vi "MU Library Demo.vi"() -> ()   [LabVIEW 2017]
uses:
  enums/MU_Interface.ctl
  enums/MU_ConfigData.ctl
  enums/MU_Param.ctl
  enums/MU_WriteVerify.ctl
  enums/MU_E2PArea.ctl
  enums/MU_Command.ctl
  enums/MU_ErrorType.ctl
  enums/MU_InterfaceInfo.ctl
  enums/MU_Error.ctl
  enums/MU_Unit.ctl
  enums/MU_AdjustmentMessage.ctl
  enums/MU_BissProfile.ctl
  Controls/MU_Functions.ctl
  handles/CalibrationHandle.ctl
  handles/CalibrationAnalyzeResultHandle.ctl
  handles/mtSyncHandle.ctl
  handles/mtSyncAnalyzeResultHandle.ctl
  MU_3SL_interface.lvlib
panel:
  in  "Stop Button":bool
  in  "TabControl":T1(tab)
  in  "MU_InterfaceInfo":T2
  in  "MU_Interface":T3
  in  "MU_Close":bool
  in  "MU_GetInterface":bool
  in  "MU_SetInterface":bool
  in  "MU_Open":bool
  out "MU_Interface":T3
  in  "MU_GetInterfaceInfo":bool caption="MU_GetInterface"
  out "information":string
  in  "interfaceOption":string
  in  "MU_ConfigData":T4
  in  "MU_ConfigData":T4
  in  "MU_GetConfig":bool
  in  "MU_SetConfig":bool
  in  "value":u32 format="0x%02x"
  out "value":u32 format="0x%02x"
  in  "MU_Initialize":bool caption="MU_GetConfig"
  in  "MU_SwitchToBiSS":bool caption="MU_GetConfig"
  out "modea":u32 format="0x%02x"
  out "modeb":u32 format="0x%02x"
  in  "MU_SwitchToBiSS_Ex":bool caption="MU_GetConfig"
  out "modea":u32 format="0x%02x"
  in  "MU_UseRevision":bool caption="MU_GetConfig"
  in  "revisionId":u32 format="0x%02x"
  in  "MU_ReadChipRevision":bool caption="MU_GetConfig"
  out "revisionId":u32 format="0x%02x"
  in  "MU_ValueOfUsedRevision":bool caption="MU_GetConfig"
  out "revisionId":u32 format="0x%02x"
  out "switched":bool
  out "isInRevision":bool
  in  "MU_Command":T5
  in  "MU_E2PArea":T6
  in  "MU_WriteVerifyEnum 2":T7 caption="MU_WriteVerify"
  in  "MU_WriteParams":bool
  in  "MU_SetParam":bool
  in  "MU_GetParam":bool
  in  "MU_ReadParams":bool
  in  "MU_ParamEnum 3":T8 caption="MU_Param"
  in  "ulValue":u64 caption="value" format="0x%08x"
  in  "MU_ParamEnum 3":T8 caption="MU_Param"
  out "pulValue":u64 caption="value" format="0x%08x"
  in  "MU_ReadStatus":bool caption="MU_GetDLLVersion"
  in  "MU_WriteEeprom":bool caption="MU_WriteParams"
  in  "MU_WriteCmdRegister":bool caption="MU_WriteParams"
  in  "MU_WriteSwitchCommand":bool caption="MU_WriteParams"
  in  "modeaNew":u32 format="0x%02x"
  in  "rplNew":u32 format="0x%02x"
  in  "MU_ReadGain":bool caption="MU_GetDLLVersion"
  in  "verify":bool
  out "valid":bool[](array[boolean])
  in  "MU_IsParameterAvailableInUsedRevision":bool caption="MU_GetParam"
  in  "MU_ParamEnum 4":T8 caption="MU_Param"
  in  "MU_ReadSens":bool caption="MU_WriteParams"
  out "data":T9 {"mt" format="0x%02x"; "st" format="0x%02x"; "err" format="0x%02x"; "warn" format="0x%02x"; "rawMaster" format="0x%02x"; "rawNonius" format="0x%02x"}
  out "noniusRawData":u16[](array[numeric])
  out "masterRawData":u16[](array[numeric])
  in  "clockFrequency":dbl
  in  "frameCycleTime":dbl
  in  "SlaveID":u32
  in  "numberOfSamples":u64
  in  "MU_acquireRawData":bool caption="MU_WriteParams"
  in  "MU_activateCalibrationConfig":bool caption="MU_WriteParams"
  in  "MU_deactivateCalibrationConfig":bool caption="MU_WriteParams"
  in  "MU_Get Calibration":bool caption="MU_WriteParams"
  in  "MU_Set Calibration":bool caption="MU_WriteParams"
  in  "MU_CreateCalibration":bool caption="MU_WriteParams"
  in  "revisionCode":u8 format="%.0x"
  in  "MU_Calibration_delete":bool caption="MU_WriteParams"
  in  "NumberOfMasterPeriods (0=autodetect)":u32
  in  "MU_Calibration_preconfigureNumberOfMasterPeriods":bool caption="MU_WriteParams"
  out "Return value":bool
  in  "noniusTrackRawData":u16[](array[numeric])
  in  "masterTrackRawData":u16[](array[numeric])
  in  "numberOfRawDataSamples":u64
  in  "MU_Calibration_analyzeRawData":bool caption="MU_WriteParams"
  in  "MU_CalibrationAnalyzeResult_delete":bool caption="MU_WriteParams"
  out "size":u64
  in  "MU_Calibration_getAnalyzeResultLog":bool caption="MU_WriteParams"
  in  "logDestSize":u64=1024
  out "logDest":string
  in  "MU_AdjustmentLogLevel":T10 format="0x%02x"
  in  "MU_Calibration_getOptimizedNoniusTrackOffsetTableBaseOnly":bool caption="MU_WriteParams"
  out "optimizedNoniusTrackOffsetTableBaseOnly":cluster{"spoBase":i8, "spoN":i8[]}
  in  "MU_Calibration_numberOfAcquiredNoniusPeriods":bool caption="MU_WriteParams"
  out "acquiredNoniusPeriods":dbl
  in  "MU_Calibration_getRelativeMasterTrackAdjustments":bool caption="MU_WriteParams"
  out "MU_Calibration_RelativeAnalogTrackAdjustments_Master":T11
  in  "MU_Calibration_getRelativeNoniusTrackAdjustments":bool caption="MU_WriteParams"
  out "MU_Calibration_RelativeAnalogTrackAdjustments_Nonius":T11
  in  "MU_Calibration_numberOfCalculatedMasterPeriods":bool caption="MU_WriteParams"
  out "CalculatedMasterPeriods":i32
  in  "MU_Calibration_isAnalogAnalysesValid":bool caption="MU_WriteParams"
  out "isAnalogAnalysesValid":bool
  in  "MU_Calibration_isNoniusAnalysesValid":bool caption="MU_WriteParams"
  out "isNoniusAnalysesValid":bool
  out "NumberOfRevolutions":dbl
  in  "MU_Calibration_numberOfRevolutions":bool caption="MU_WriteParams"
  in  "MU_Calibration_numberOfAcquiredMasterPeriods":bool caption="MU_WriteParams"
  out "acquiredMasterPeriods":dbl
  in  "MU_Calibration_minimalNumberOfSamplesPerMasterPeriod":bool caption="MU_WriteParams"
  out "minimalNumberOfSamplesPerMasterPeriod":dbl
  in  "MU_Calibration_getOptimizedNoniusTrackOffsetTable":bool caption="MU_WriteParams"
  out "optimizedNoniusTrackOffsetTable":cluster{"spoBase":i8, "spoN":i8[]}
  in  "MU_Calibration_noniusTrackOffsetCurve":bool caption="MU_WriteParams"
  out "TrackOffset":i32[](array[numeric])
  in  "MU_Calibration_noniusPhaseMargin":bool caption="MU_WriteParams"
  out "PhaseMargin":i32[](array[numeric])
  out "PhaseError":i32[](array[numeric])
  in  "MU_Calibration_noniusPhaseError":bool caption="MU_WriteParams"
  out "Return Value":u64
  out "SingleturnPosition":dbl[](array[numeric])
  in  "Continuous":bool
  in  "MU_Calibration_calculateNoniusPosition":bool caption="MU_WriteParams"
  in  "MU_Unit":T12 format="0x%02x"
  out "NoniusPhaseMarginMin":i32
  in  "MU_Calibration_noniusPhaseMarginMin":bool caption="MU_WriteParams"
  in  "MU_Calibration_noniusPhaseMarginMax":bool caption="MU_WriteParams"
  out "NoniusPhaseMarginMax":i32
  in  "MU_Calibration_noniusPhaseRangeLimit":bool caption="MU_WriteParams"
  in  "MU_Calibration_noniusUpperPhaseMargin":bool caption="MU_WriteParams"
  in  "MU_Calibration_NoniusLowerPhaseMargin":bool caption="MU_WriteParams"
  out "noniusLowerPhaseMargin":dbl
  out "noniusUpperPhaseMargin":dbl
  out "noniusPhaseRangeLimit":i32
  out "NumberOfNoniusCurveSamples":u64
  in  "MU_Calibration_numberOfNoniusCurveSamples":bool caption="MU_WriteParams"
  in  "optimizedNoniusTrackOffsetTable":cluster{"spoBase":i8, "spoN":i8[]}={"spoBase"=0, "spoN"=[0, 0, 0, 0, 0, 0, 0, 0, 0, 0, 0, 0, 0, 0, 0, 0]}
  in  "MU_Calibration_setCurrentNoniusTrackOffsetTable":bool caption="MU_WriteParams"
  in  "noniusAdjustments":T13 {"phaseRange" format="%.0x"; "phase" format="%.0x"; "cosineOffset" format="%.0x"; "sineOffset" format="%.0x"; "cosineGain" format="%.0x"}
  in  "masterAdjustments":T13 {"phaseRange" format="%.0x"; "phase" format="%.0x"; "cosineOffset" format="%.0x"; "sineOffset" format="%.0x"; "cosineGain" format="%.0x"}
  in  "MU_Calibration_setCurrentAnalogTrackAdjustments":bool caption="MU_WriteParams"
  out "function return":bool
  in  "MU_Calibration_adjustAnalogByAnalyzeResult":bool caption="MU_WriteParams"
  in  "MU_AdjustmentLogLevel":T10 format="0x%02x"
  out "Result":bool
  out "adjustMessage":string
  in  "adjustmentMessageBufferSize":u64=1024
  in  "MU_Calibration_isAnalogAnalyzeResultAdjustable":bool caption="MU_WriteParams"
  in  "MU_Calibration_getAnalogMasterTrackAdjustments":bool caption="MU_WriteParams"
  out "masterAdjustments":T13 {"phaseRange" format="%.0x"; "phase" format="%.0x"; "cosineOffset" format="%.0x"; "sineOffset" format="%.0x"; "cosineGain" format="%.0x"}
  in  "MU_Calibration_getAnalogNoniusTrackAdjustments":bool caption="MU_WriteParams"
  out "noniusAdjustments":T13 {"phaseRange" format="%.0x"; "phase" format="%.0x"; "cosineOffset" format="%.0x"; "sineOffset" format="%.0x"; "cosineGain" format="%.0x"}
  in  "MU_Calibration_getNoniusTrackOffsetTable":bool caption="MU_WriteParams"
  out "NoniusTrackOffsetTable":cluster{"spoBase":i8, "spoN":i8[]}
  out "noniusTrackOffsetTable":cluster{"spoBase":i8, "spoN":i8[]}
  in  "noniusTrackOffsetTableParameters":cluster{"spoBase":u8, "spoN":u8[]}={"spoBase"=0, "spoN"=[0, 0, 0, 0, 0, 0, 0, 0, 0, 0, 0, 0, 0, 0, 0, 0]}
  out "noniusTrackOffsetTableParameters":cluster{"spoBase":u8, "spoN":u8[]}
  in  "noniusTrackOffsetTable":cluster{"spoBase":i8, "spoN":i8[]}={"spoBase"=0, "spoN"=[0, 0, 0, 0, 0, 0, 0, 0, 0, 0, 0, 0, 0, 0, 0, 0]}
  in  "MU_getNoniusTrackOffsetTableParameters":bool caption="MU_WriteParams"
  in  "MU_getNoniusTrackOffsetTableByParameters":bool caption="MU_WriteParams"
  out "nextClockFrequency":dbl format="%#_6f"
  in  "clockFrequency_hz":dbl format="%#_6f"
  in  "MU_Interface_nextPossibleClockFreq":bool caption="MU_WriteParams"
  in  "frameCycleTime_s":dbl format="%#_6f"
  in  "MU_Interface_nextPossibleFrameCycleTime":bool caption="MU_WriteParams"
  out "nextFrameCycleTime":dbl format="%#_6f"
  out "nearestFrameCycleTime":dbl format="%#_6f"
  in  "frameCycleTime_s":dbl format="%#_6f"
  in  "MU_Interface_nearestPossibleFrameCycleTime":bool caption="MU_WriteParams"
  out "nearestClockFrequency":dbl format="%#_6f"
  in  "clockFrequency_hz":dbl format="%#_6f"
  in  "MU_Interface_nearestPossibleClockFreq":bool caption="MU_WriteParams"
  in  "MU_Interface":T3 format="0x%02x"
  in  "MU_Interface":T3 format="0x%02x"
  in  "MU_Interface":T3 format="0x%02x"
  in  "MU_Interface":T3 format="0x%02x"
  in  "MU_acquire3TrackMtSyncData":bool caption="MU_WriteParams"
  in  "Samples":u64
  out "SyncData":T14(array[cluster])
  in  "MU_acquireMtSyncData":bool caption="MU_WriteParams"
  in  "Samples":u64
  out "data":T15(array[cluster])
  in  "MU_activateMtSyncConfig":bool caption="MU_WriteParams"
  in  "MU_deactivateMtSyncConfig":bool caption="MU_WriteParams"
  in  "MU_activate3TrackMtSyncConfig":bool caption="MU_WriteParams"
  in  "MU_deactivate3TrackMtSyncConfig":bool caption="MU_WriteParams"
  in  "MU_MtSync_calculatePosition":bool caption="MU_WriteParams"
  in  "SyncData":T15(array[cluster])
  out "MT_Position":dbl[](array[numeric])
  in  "Samples":u64
  in  "MtTrackOffset":u8
  in  "Calibration Unit":u32
  in  "resolution":u64
  in  "Continuous (F)":bool
  in  "MU_getMtSync":bool caption="MU_WriteParams"
  in  "MU_updateMtSync":bool caption="MU_WriteParams"
  in  "mtMovementIsReverse":bool
  in  "nMtSyncBits":u64
  in  "MU_createMtSync":bool caption="MU_WriteParams"
  in  "MU_MtSync_delete":bool caption="MU_WriteParams"
  in  "numberOfSamples":u64
  in  "data":T15(array[cluster])
  in  "MU_MtSync_analyzeData":bool caption="MU_WriteParams"
  in  "MU_MtAnalyzeResult_delete":bool caption="MU_WriteParams"
  out "optimalSpoMt":u8
  in  "MU_MtAnalyzeResult_optimalSpoMt":bool caption="MU_WriteParams"
  in  "MtTrackOffset":u8
  out "MT_OffsetError":dbl[](array[numeric])
  in  "MU_MtAnalyzeResult_calculateOffsetError":bool caption="MU_WriteParams"
  in  "Samples":u64
  out "Return Value":u64
  out "UpperOffsetErrorMargin":dbl
  in  "MtTrackOffset":u8
  in  "MU_MtAnalyzeResult_upperOffsetErrorMargin":bool caption="MU_WriteParams"
  in  "MtTrackOffset":u8
  out "LowerOffsetErrorMargin":dbl
  in  "MU_MtAnalyzeResult_lowerOffsetErrorMargin":bool caption="MU_WriteParams"
  out "OffsetErrorRangeLimit":dbl
  in  "MU_MtAnalyzeResult_offsetErrorRangeLimit":bool caption="MU_WriteParams"
  out "MinOffsetError":dbl
  in  "MtTrackOffset":u8
  in  "MU_MtAnalyzeResult_minOffsetError":bool caption="MU_WriteParams"
  in  "MtTrackOffset":u8
  out "MaxOffsetError":dbl
  in  "MU_MtAnalyzeResult_maxOffsetError":bool caption="MU_WriteParams"
  in  "MU_BissProfile":T16 format="0x%02x"
  in  "MU_generateBissProfileId":bool caption="MU_GetDLLVersion"
  in  "MU_generateBissIdentifier":bool caption="MU_GetDLLVersion"
  out "MU_Error":T17
  in  "MU_SaveParams":bool
  in  "MU_LoadParams":bool
  in  "data":u32 format="0x%02x"
  in  "MU_SPIActivate":bool caption="MU_GetDLLVersion"
  in  "MU_GetLastError":bool caption="MU_GetDLLVersion"
  out "lastErrorText":string
  out "MU_ErrorType":T18
  in  "MU_CalcPres_POS":bool caption="MU_GetDLLVersion"
  in  "value":u64 format="0x%08x"
  in  "MU_GetPres_POS":bool caption="MU_GetDLLVersion"
  out "value":u64 format="0x%08x"
  in  "MU_WriteVerifyEnum":T7 caption="MU_WriteVerify"
  out "modea":u32 format="0x%02x"
  in  "MU_EnableGetMT":bool caption="MU_GetDLLVersion"
  in  "MU_DisableGetMT":bool caption="MU_GetDLLVersion"
  in  "pcCfgFilename":path caption="filepath"
  in  "pcCfgFilename 2":path caption="filepath"
  out "switched":bool
  in  "MU_ReadChipRevisionOfParameterFile":bool caption="MU_SaveParams"
  in  "pcCfgFilename 5":path caption="filepath"
  out "revisionCode":u32 format="0x%02x"
  out "bissProfileId":u16 format="%.0x"
  out "deviceID":u64 format="%.0x"
  out "mfgID":u16 format="%.0x"
  out "versionBuild":u16 format="%.0x"
  out "versionPatch":u16 format="%.0x"
  out "versionMinor":u16 format="%.0x"
  out "versionMajor":u16 format="%.0x"
  out "versionSuffixString":string
  in  "MU_GetVersionSuffixString":bool caption="MU_WriteParams"
  in  "MU_GetVersionBuild":bool caption="MU_WriteParams"
  in  "MU_GetVersionPatch":bool caption="MU_WriteParams"
  in  "MU_GetVersionMinor":bool caption="MU_WriteParams"
  in  "MU_GetVersionMajor":bool caption="MU_WriteParams"
  out "versionString":string
  in  "MU_GetVersionString":bool caption="MU_WriteParams"
  out "version":u32[](array[numeric]) format="0x%02x"
  in  "MU_GetDLLVersion":bool
  in  "MU_GetRegister":bool
  in  "MU_SetRegister":bool
  in  "address":u32 format="0x%02x"
  in  "ulValue":u32 caption="value" format="0x%02x"
  in  "MU_WriteVerifyEnum 2":T7 caption="MU_WriteVerify"
  in  "ulAdr":u32 caption="address" format="0x%02x"
  out "pulValue":u32 caption="value" format="0x%02x"
  in  "MU_WriteRegister":bool caption="MU_GetRegister"
  in  "address":u32 format="0x%02x"
  in  "count":u32 format="0x%02x"
  in  "values":u32[](array[numeric]) format="0x%02x"
  in  "MU_ReadRegister":bool caption="MU_GetRegister"
  in  "address":u32 format="0x%02x"
  in  "count":u32 format="0x%02x"
  out "values":u32[](array[numeric]) format="0x%02x"
  in  "MU_SaveRegister":bool caption="MU_SaveParams"
  in  "address":u32 format="0x%02x"
  in  "count":u32 format="0x%02x"
  in  "values":u32[](array[numeric]) format="0x%02x"
  in  "MU_LoadRegister":bool caption="MU_LoadParams"
  in  "count":u32 format="0x%02x"
  in  "address":u32 format="0x%02x"
  out "values":u32[](array[numeric]) format="0x%02x"
  in  "values":u32[](array[numeric]) format="0x%02x"
  in  "count":u32 format="0x%02x"
  in  "address":u32 format="0x%02x"
  in  "MU_WriteRegisterSSI":bool caption="MU_GetRegister"
  in  "pcFilename":path caption="filepath"
  in  "pcCfgFilename 3":path caption="filepath"
  in  "MU_WriteRegister_I2C":bool caption="MU_GetDLLVersion"
  in  "values":u32[](array[numeric]) format="0x%02x"
  in  "MU_WriteRegister_I2C_Ex":bool caption="MU_GetDLLVersion"
  in  "values":u32[](array[numeric]) format="0x%02x"
  in  "i2cSlaveAddress":u32 format="0x%02x"
  in  "registerCount":u32 format="0x%02x"
  in  "registerCount":u32 format="0x%02x"
  in  "registerAddress":u32 format="0x%02x"
  in  "i2cSlaveAddress":u32 format="0x%02x"
  in  "MU_ReadRegister_I2C":bool caption="MU_GetDLLVersion"
  out "values":u32[](array[numeric]) format="0x%02x"
  in  "i2cSlaveAddress":u32 format="0x%02x"
  in  "registerCount":u32 format="0x%02x"
  in  "registerAddress":u32 format="0x%02x"
  in  "MU_LoadRegisterEx":bool caption="MU_GetDLLVersion"
  out "values":u32[](array[numeric]) format="0x%02x"
  in  "registerCount":u32 format="0x%02x"
  in  "MU_SaveRegisterEx":bool caption="MU_GetDLLVersion"
  in  "values":u32[](array[numeric]) format="0x%02x"
  in  "registerCount":u32 format="0x%02x"
  in  "registerAddress":u32 format="0x%02x"
  in  "pcCfgFilename 4":path caption="filepath"
  in  "pcFilename 2":path caption="filepath"
  in  "valid":bool[](array[boolean])
  out "valid":bool[](array[boolean])
  # "iC-MU Series Library Demo"
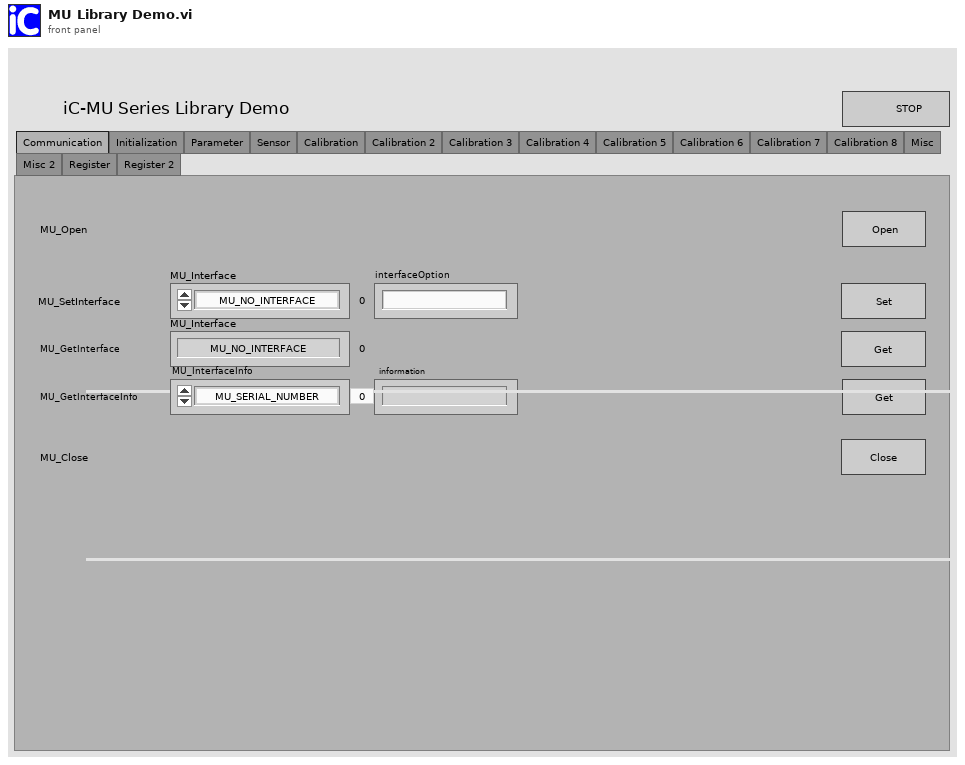
[diagram p1: front panel]
types:
  T1 = enum32{"Communication", "Initialization", "Parameter", "Sensor", "Calibration", "Calibration 2", "Calibration 3", "Calibration 4", "Calibration 5", "Calibration 6", "Calibration 7", "Calibration 8", "Misc", "Misc 2", "Register", "Register 2"}
  T2 = typedef "MU_3SL_interface.lvlib/MU_InterfaceInfo.ctl" = enum32{"MU_SERIAL_NUMBER", "MU_DRIVER_VERSION"}
  T3 = typedef "MU_3SL_interface.lvlib/MU_Interface.ctl" = enum32{"MU_NO_INTERFACE", "MU_MB3U_SPI", "MU_MB3U_BISS", "MU_MB4U", "MU_MB5U"}
  T4 = typedef "MU_3SL_interface.lvlib/MU_ConfigData.ctl" = enum32{"MU_RESERVED0", "MU_FREQ_SPI", "MU_MASTERVER", "MU_MASTERREV", "MU_SLAVE_ID", "MU_FREQ_SCD", "MU_CLKENI", "MU_FREQ_AGS", "MU_SLAVE_COUNT", "MU_START_CONTROL_FRAME", "MU_REG_END", "MU_FREQ_SSI", "MU_READ_STATUS_ENABLE", "MU_USB_PERFORMANCE", "MU_READ_GAIN_ENABLE", "MU_BP", "MU_UPDATE_BISSID_ENABLE", "MU_ENABLE_TTL"}
  T5 = typedef "MU_3SL_interface.lvlib/MU_Command.ctl" = enum32{"MU_CMD_NO_FUNCTION", "MU_CMD_WRITE_ALL", "MU_CMD_WRITE_OFF", "MU_CMD_ABS_RESET", "MU_CMD_NON_VER", "MU_CMD_MT_RESET", "MU_CMD_MT_VER", "MU_CMD_SOFT_RESET", "MU_CMD_SOFT_PRES", "MU_CMD_SOFT_E2P_PRES", "MU_CMD_I2C_COM", "MU_CMD_EVENT_COUNT", "MU_CMD_SWITCH", "MU_CMD_CRC_VER", "MU_CMD_CRC_CALC", "MU_CMD_SET_MTC", "MU_CMD_RES_MTC", "MU_CMD_RESERVED0", "MU_CMD_MODEA_SPI", "MU_CMD_ROT_POS", "MU_CMD_ROT_POS_E2P"}
  T6 = typedef "MU_3SL_interface.lvlib/MU_E2PArea.ctl" = enum32{"MU_E2P_CFG"}
  T7 = typedef "MU_3SL_interface.lvlib/MU_WriteVerify.ctl" = enum32{"MU_SETONLY", "MU_WRITE", "MU_VERIFY"}
  T8 = typedef "MU_3SL_interface.lvlib/MU_Param.ctl" = enum32{"MU_GF_M", "MU_GC_M", "MU_GX_M", "MU_VOSS_M", "MU_VOSC_M", "MU_PH_M", "MU_PHR_M", "MU_CIBM", "MU_ENAC", "MU_GF_N", "MU_GC_N", "MU_GX_N", "MU_VOSS_N", "MU_VOSC_N", "MU_PH_N", "MU_PHR_N", "MU_MODEA", "MU_NTOA", "MU_MODEB", "MU_CFGEW", "MU_EMTD", "MU_ACRM_RES", "MU_NCHK_NON", "MU_NCHK_CRC", "MU_ACC_STAT", "MU_FILT", "MU_LIN", "MU_ESSI_MT", "MU_ROT_MT", "MU_MPC", "MU_SPO_MT", "MU_MODE_MT", "MU_SBL_MT", "MU_CHK_MT", "MU_GET_MT", "MU_OUT_MSB", "MU_OUT_ZERO", "MU_OUT_LSB", "MU_MODE_ST", "MU_RSSI", "MU_GSSI", "MU_RESABZ", "MU_FRQAB", "MU_ENIF_AUTO", "MU_SS_AB", "MU_ROT_ALL", "MU_INV_Z", "MU_INV_B", "MU_INV_A", "MU_PP60UVW", "MU_CHYS_AB", "MU_LENZ", "MU_PPUVW", "MU_RPL", "MU_TEST", "MU_ROT_POS", "MU_OFF_ABZ", "MU_OFF_POS", "MU_OFF_COM", "MU_PA0_CONF", "MU_AFGAIN_M", "MU_ACGAIN_M", "MU_AFGAIN_N", "MU_ACGAIN_N", "MU_EDSBANK", "MU_PROFILE_ID", "MU_SERIAL", "MU_OFF_UVW", "MU_PRES_POS", "MU_SPO_BASE", "MU_SPO_0", "MU_SPO_1", "MU_SPO_2", "MU_SPO_3", "MU_SPO_4", "MU_SPO_5", "MU_SPO_6", "MU_SPO_7", "MU_SPO_8", "MU_SPO_9", "MU_SPO_10", "MU_SPO_11", "MU_SPO_12", "MU_SPO_13", "MU_SPO_14", "MU_SPO_15", "MU_RPL_RESET", "MU_I2C_DEV_START", "MU_I2C_RAM_START", "MU_I2C_RAM_END", "MU_I2C_DEVID", "MU_I2C_RETRY", "MU_HARD_REV", "MU_DEV_ID0", "MU_DEV_ID1", "MU_DEV_ID2", "MU_DEV_ID3", "MU_DEV_ID4", "MU_DEV_ID5", "MU_MFG_ID0", "MU_MFG_ID1", "MU_CRC16", "MU_CRC8", "MU_AM_MIN", "MU_AM_MAX", "MU_AN_MIN", "MU_AN_MAX", "MU_STUP", "MU_CMD_EXE", "MU_FRQ_CNV", "MU_FRQ_ABZ", "MU_NON_CTR", "MU_MT_CTR", "MU_MT_ERR", "MU_EPR_ERR", "MU_CRC_ERR"}
  T9 = cluster{"mt":u32, "st":u32, "err":u32, "warn":u32, "rawMaster":u32, "rawNonius":u32}
  T10 = typedef "MU_3SL_interface.lvlib/MU_AdjustmentMessage.ctl" = enum32{"MU_LOG_NONE", "MU_LOG_ERRORS", "MU_LOG_WARNINGS", "MU_LOG_ERRORS_WARNINGS", "MU_LOG_NOTE", "MU_LOG_ERRORS_NOTE", "MU_LOG_WARNINGS_NOTE", "MU_LOG_ALL"}
  T11 = cluster{"cosineGain_lsb":dbl, "sineOffset_lsb":dbl, "cosineOffset_lsb":dbl, "phase_lsb":dbl}
  T12 = typedef "MU_3SL_interface.lvlib/MU_Unit.ctl" = enum32{"MU_RESOLUTION", "MU_TURN", "MU_DEGREE", "MU_RAD"}
  T13 = cluster{"cosineGain":u8, "sineOffset":u8, "cosineOffset":u8, "phase":u8, "phaseRange":u8}
  T14 = cluster{"SingleTurnPosition":u32, "InternalSingleTurnPosition":u32, "NormalizedExternalMultiTurnSyncBits":u32, "NormalizedInternalMultiTurnSyncBits":u32, "externalMultiTurnPosition":u32, "multiTurnPosition":u32, "scdDataH":u64}[]
  T15 = cluster{"SingleTurnPosition":u32, "InternalSingleTurnPosition":u32, "NormalizedExternalMultiTurnSyncBits":u32, "NormalizedInternalMultiTurnSyncBits":u32, "externalMultiTurnPosition":u32, "multiTurnPosition":u32, "scdData":u64}[]
  T16 = typedef "MU_3SL_interface.lvlib/MU_BissProfile.ctl" = enum32{"MU_BISS_PROFILE_BP1", "MU_BISS_PROFILE_BP3"}
  T17 = typedef "MU_3SL_interface.lvlib/MU_Error.ctl" = enum32{"MU_OK", "MU_INVALID_HANDLE", "MU_INTERFACEDRIVER_NOT_FOUND", "MU_INTERFACE_NOT_FOUND", "MU_INVALID_INTERFACE", "MU_NO_INTERFACE_SELECTED", "MU_INVALID_PARAMETER", "MU_INVALID_ADDRESS", "MU_INVALID_VALUE", "MU_USB_ERROR", "MU_FILE_NOT_FOUND", "MU_INVALID_FILE", "MU_SPI_ERROR", "MU_SPI_DISMISS", "MU_SPI_FAIL", "MU_SPI_BUSY_TIMEOUT", "MU_VERIFY_FAILED", "MU_MASTERCOMM_FAILED", "MU_BISSCOMM_FAILED", "MU_INVALID_BISSMASTER", "MU_USB_HIGHSPEED_WARNING", "MU_FAST_ROTATION", "MU_SLOW_ROTATION", "MU_FILE_ACCESS_DENIED", "MU_READPARAM_SSI", "MU_SSIRING_ERROR", "MU_SEMI_ROTATION", "MU_BISS_REGERROR", "MU_INTERNAL_CALIB_ERROR", "MU_INVALID_CONFIGURATION", "MU_CALIBRATION_FAILED", "MU_ACQUISITION_FAILED", "MU_GAIN_LIMIT", "MU_OFFSET_LIMIT", "MU_PHASE_LIMIT", "MU_BAD_CAL_DATA", "MU_I2C_COMM_FAILED", "MU_USB_DATA_LOSS", "MU_MT_SYNC_FAILED", "MU_UNKNOWN_ERROR", "MU_UNKNOWN_REVISION", "MU_UNSUPPORTED_REVISION", "MU_UNKNOWN_PARAMETER", "MU_PARAMETER_NOT_IN_REVISION", "MU_REVISION_NOT_SET", "MU_UNSUPPORTED_CHIP", "MU_CONTRADICTORY_REVISIONS", "MU_FRAME_RATE_NOT_SUPPORTED", "MU_CLOCK_FREQUENCY_NOT_SUPPORTED", "MU_FRAME_CYCLE_TIME_TO_SHORT", "MU_NO_BISS_PROFILE_ID"}
  T18 = typedef "MU_3SL_interface.lvlib/MU_ErrorType.ctl" = enum32{"MU_NONE", "MU_HINT", "MU_WARNING", "MU_PROGRAMMING_ERROR", "MU_OPERATING_ERROR", "MU_COMMUNICATION_ERROR"}
  T19 = typedef "MU_3SL_interface.lvlib/mtSyncAnalyzeResultHandle.ctl" = u64
  T20 = typedef "MU_3SL_interface.lvlib/mtSyncHandle.ctl" = u64
  T21 = typedef "MU_3SL_interface.lvlib/CalibrationAnalyzeResultHandle.ctl" = u64
  T22 = typedef "MU_3SL_interface.lvlib/CalibrationHandle.ctl" = u64
  T23 = typedef "MU_Functions.ctl" = enum16{"Start Demo", "Open", "Close", "Set Interface", "Get Interface", "Set Config", "Get Config", "Switch to BiSS", "Switch to BiSS Ex", "Enable Get MT", "Disable Get MT", "Initialize", "Set Param", "Get Param", "Is Parameter Available In Used Revision", "Write Params", "Read Params", "Read Status", "Read Gain", "Write Eeprom", "Write Cmd Register", "Write Switch Command", "Read Sens", "Get Calibration", "Set Calibration", "Calibration_createCalibration", "Calibration_getAnalyzeResultLog", "Calibration_minimalNumberOfSamplesPerMasterPeriod", "Calibration_noniusPhaseRangeLimit", "Calibration_noniusUpperPhaseMargin", "Calibration_noniusLowerPhaseMargin", "Calibration_getAnalogMasterTrackAdjustments", "Calibration_getAnalogNoniusTrackAdjustments", "Calibration_getNoniusTrackOffsetTable", "Calibration_isAnalogAnalysesValid", "Calibration_isNoniusAnalysesValid", "getNoniusTrackOffsetTableParameters", "getNoniusTrackOffsetTableByParameters", "createMtSync", "getVersionMajor", "getVersionMinor", "getVersionPatch", "getVersionBuild", "getVersionSuffixString", "Calibration_setCurrentAnalogTrackAdjustments", "ActivateCalibrationConfig", "DeactivateCalibrationConfig", "InterfaceNearestPossibleClockFreq", "InterfaceNearestPossibleFrameCycleTime", "InterfaceNextPossibleFrameCycleTime", "InterfaceNextPossibleClockFreq", "generateBissIdentifier", "generateBissProfileId", "AcquireRawData", "Calibration_AnalyzeRawData", "Calibration_GetRelativeMasterTrackAdjustments", "Calibration_GetRelativeNoniusTrackAdjustment", "Calibration_AdjustAnalogByAnalyzeResult", "Calibration_AnalyzeResultdelete", "Calibration_delete", "Calibration_NumberOfCalculatedMasterPeriods", "Calibration_NumberOfNoniusCurveSamples", "Calibration_NoniusPhaseError", "Calibration_NoniusTrackOffsetCurve", "Calibration_NoniusPhaseMargin", "Calibration_GetOptimizedNoniusTrackOffsetTable", "Calibration_GetOptimizedNoniusTrackOffsetBaseOnly", "Calibration_SetCurrentNoniusTrackOffsetTable", "Calibration_PreconfigureNumberOfMasterPeriods", "Calibration_NoniusPhaseMarginMax", "Calibration_NoniusPhaseMarginMin", "Calibration_IsAnalogAnalyzeResultAdjustable", "Calibration_NumberOfAcquiredMasterPeriods", "Calibration_NumberOfAcquiredNoniusPeriods", "ActivateMtSyncConfig", "AcquireMtSyncData", "DeactivateMtSyncConfig", "GetMtSync", "MtSync_analyzeData", "MtAnalyzeResult_optimalSpoMt", "UpdateMtSync", "MtAnalyzeResult_delete", "MtSync_delete", "Activate3TrackMtSyncConfig", "Acquire3TrackMtSyncData", "Deactivate3TrackMtSyncConfig", "MtAnalyzeResult_calculateOffsetError", "Calibration_calculateNoniusPosition", "MtSync_calculatePosition", "MtAnalyzeResult_maxOffsetError", "MtAnalyzeResult_minOffsetError", "MtAnalyzeResult_offsetErrorRangeLimit", "MtAnalyzeResult_lowerOffsetErrorMargin", "MtAnalyzeResult_upperOffsetErrorMargin", "Calibration_numberOfRevolutions", "Save Params", "Read Chip Revision Of Parameter File", "Load Params", "Get Last Error", "Get DLL Version", "Calc PRES_POS", "Get PRES_POS", "Use Revision", "Value Of Used Revision", "Read Chip Revision", "Set Register", "Get Register", "Write Register", "Read Register", "Write Register SSI", "Save Register", "Load Register", "Spi Activate", "Get Interface Info", "Write Register I2C", "Write Register I2C Ex", "Read Register I2C", "Save Register Ex", "Load Register Ex", "Get Version String", "Stop Demo"}
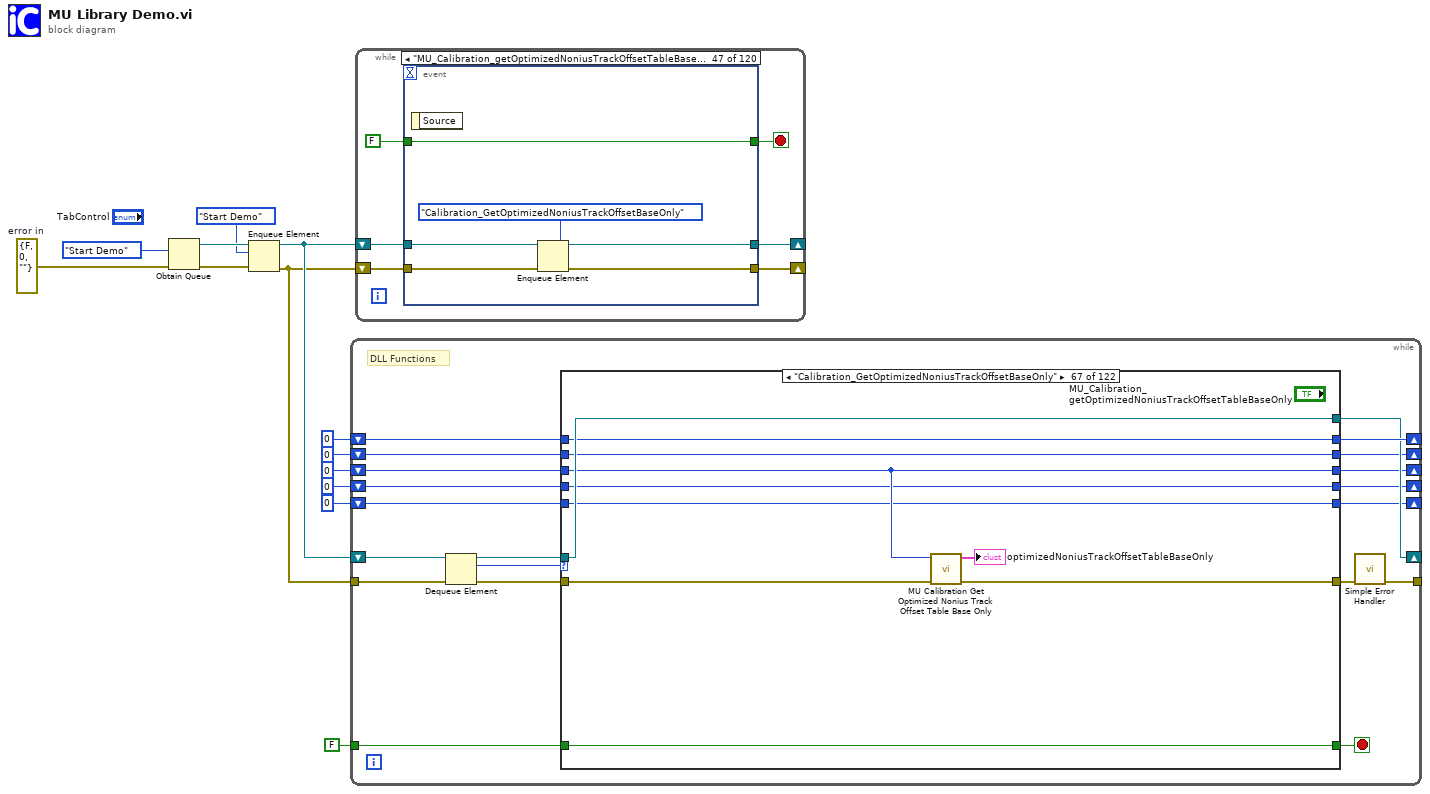
[diagram p0: block diagram]
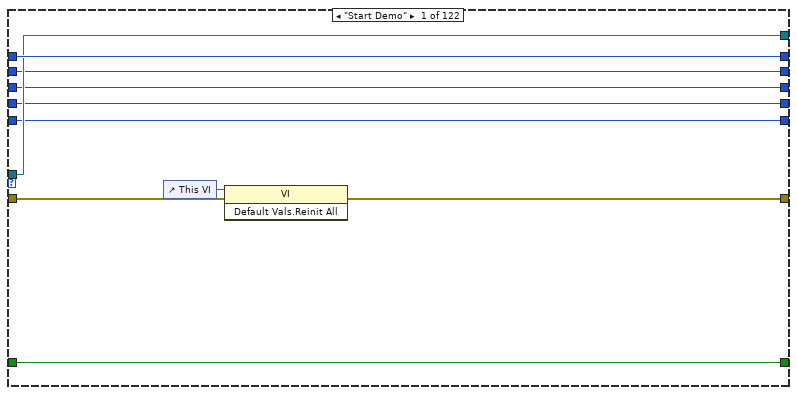
[diagram p2: hidden frame]
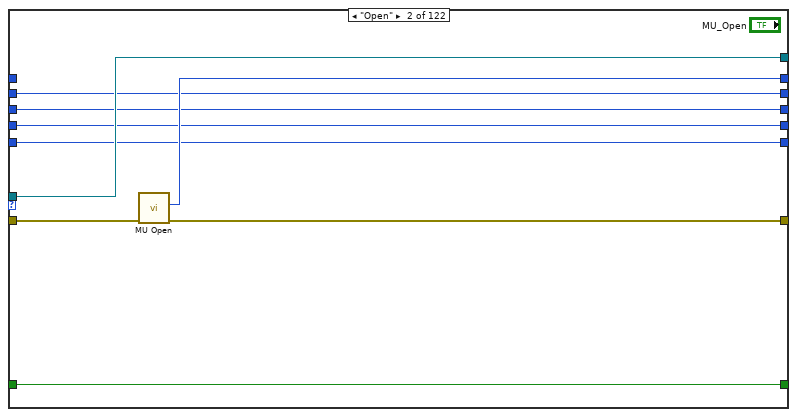
[diagram p3: hidden frame]
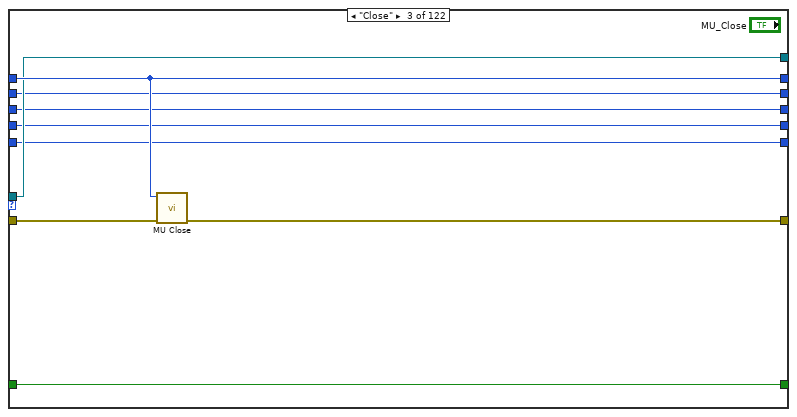
[diagram p4: hidden frame]
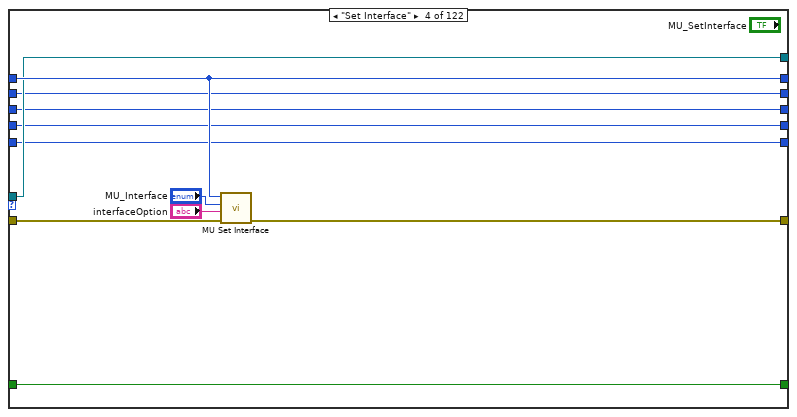
[diagram p5: hidden frame]
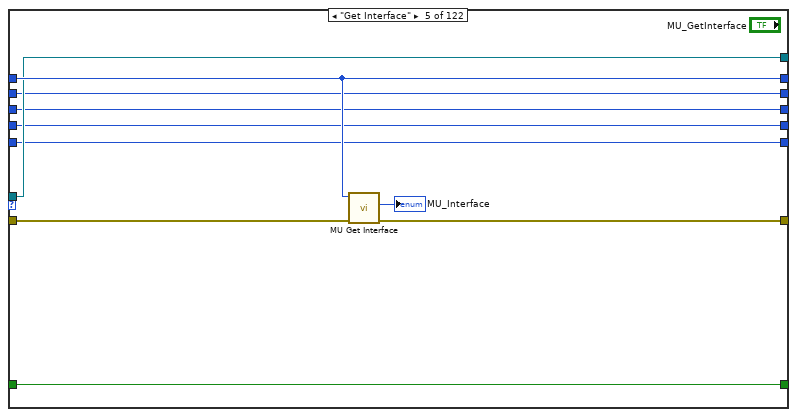
[diagram p6: hidden frame]
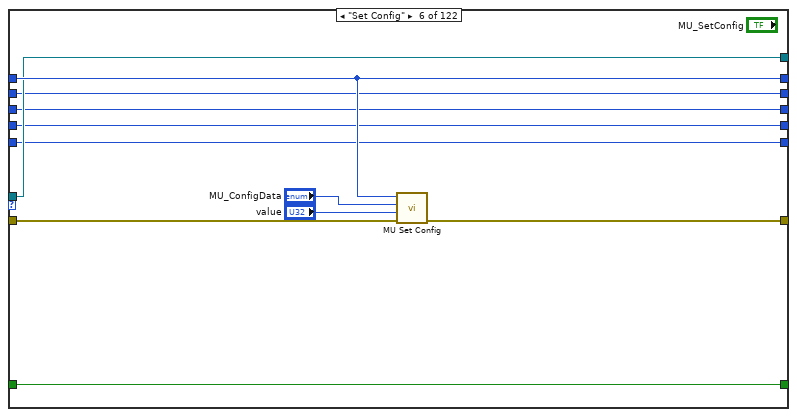
[diagram p7: hidden frame]
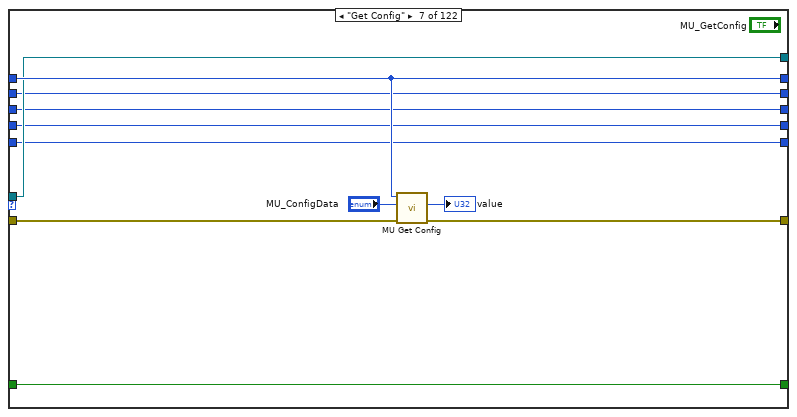
[diagram p8: hidden frame]
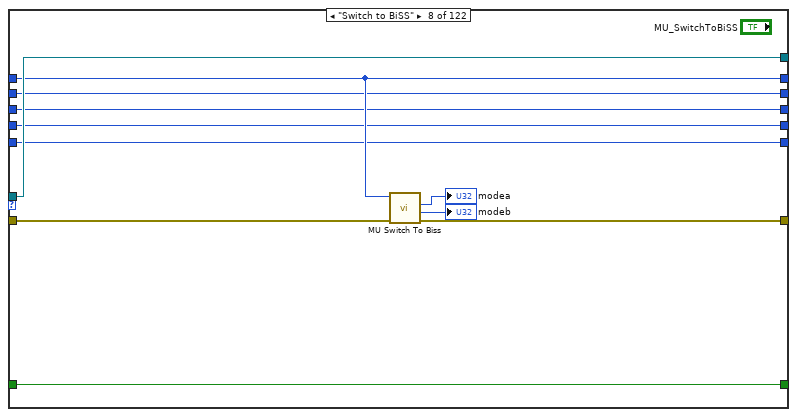
[diagram p9: hidden frame]
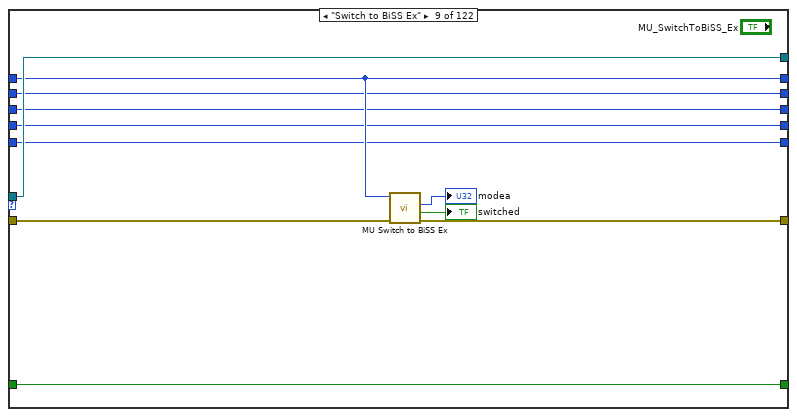
[diagram p10: hidden frame]
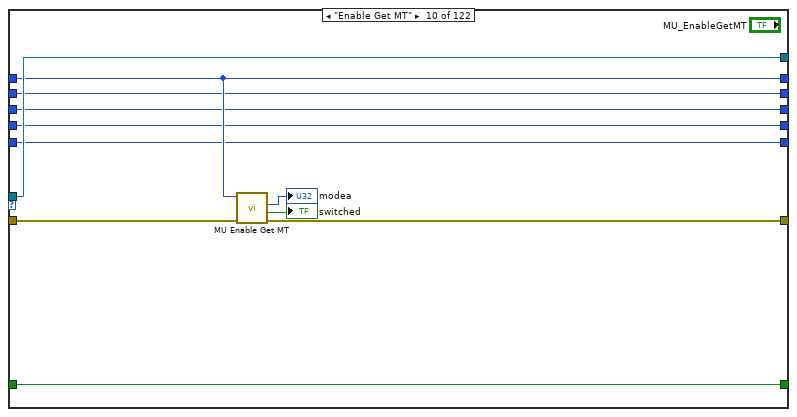
[diagram p11: hidden frame]
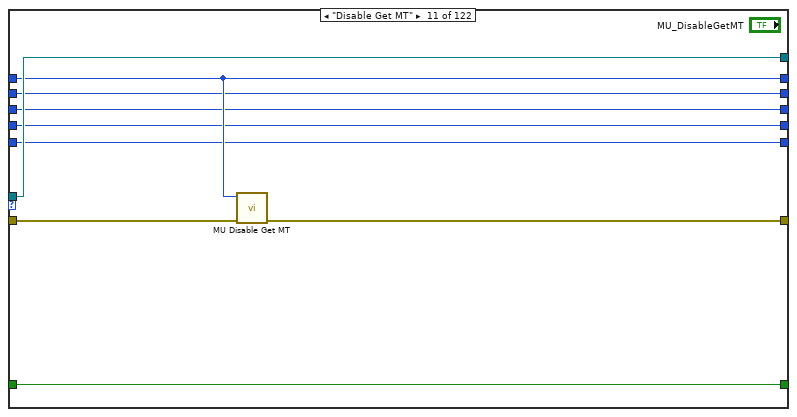
[diagram p12: hidden frame]
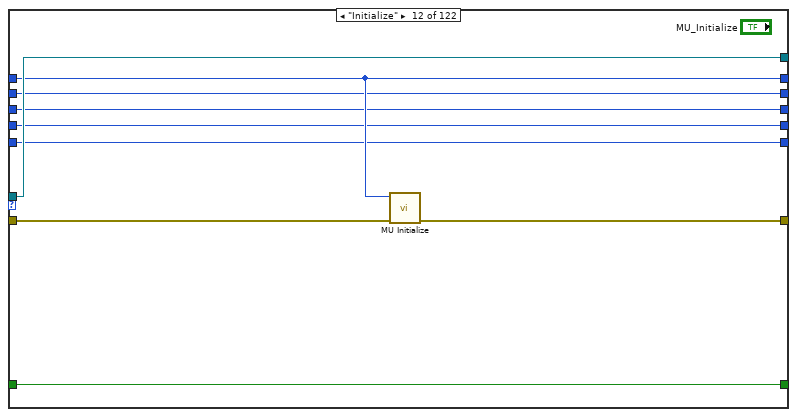
[diagram p13: hidden frame]
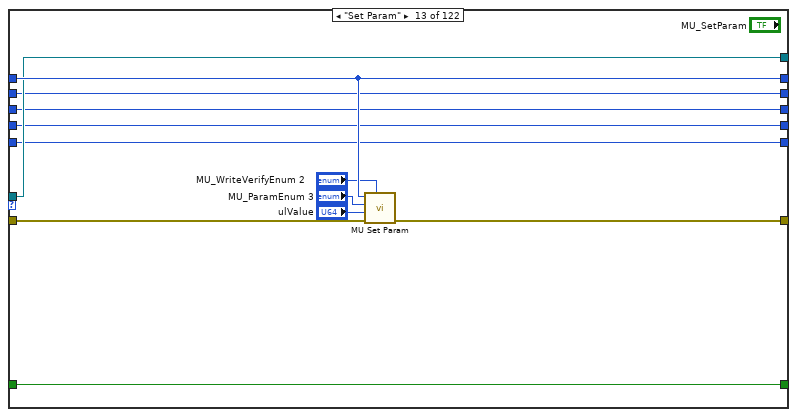
[diagram p14: hidden frame]
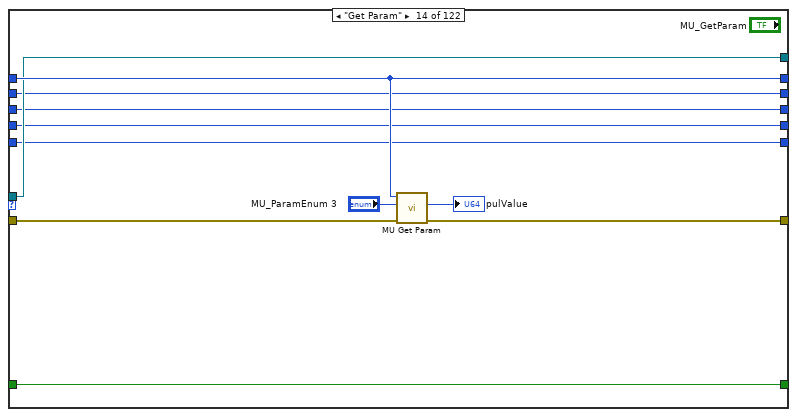
[diagram p15: hidden frame]
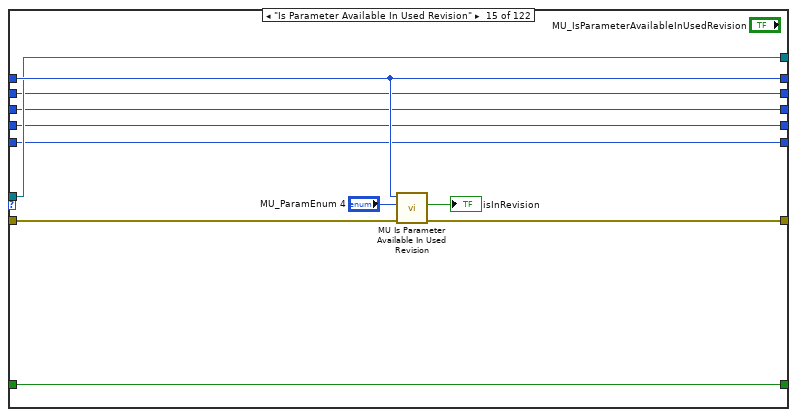
[diagram p16: hidden frame]
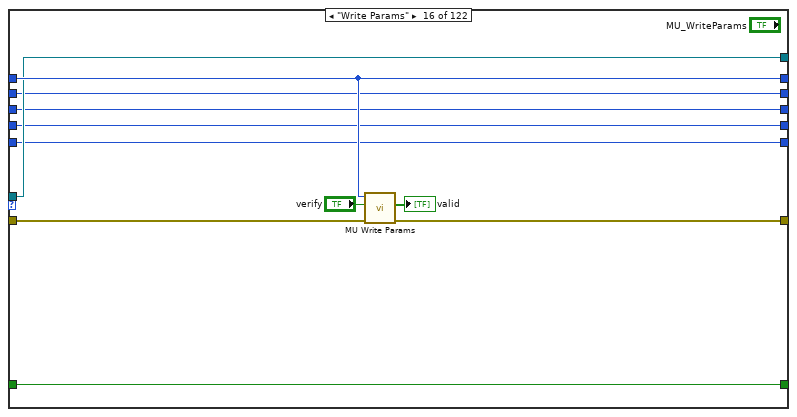
[diagram p17: hidden frame]
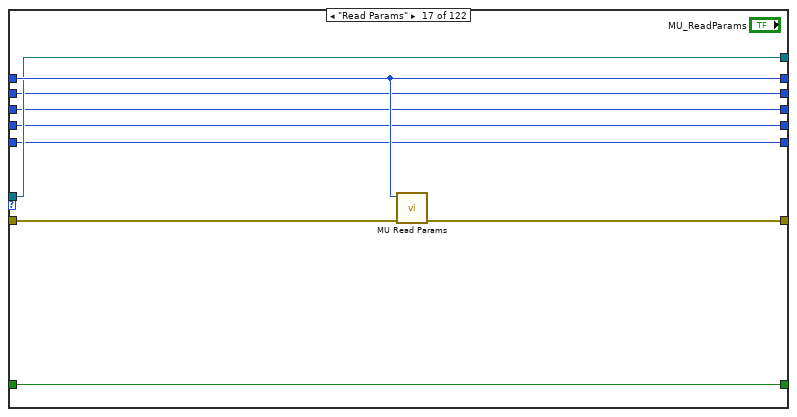
[diagram p18: hidden frame]
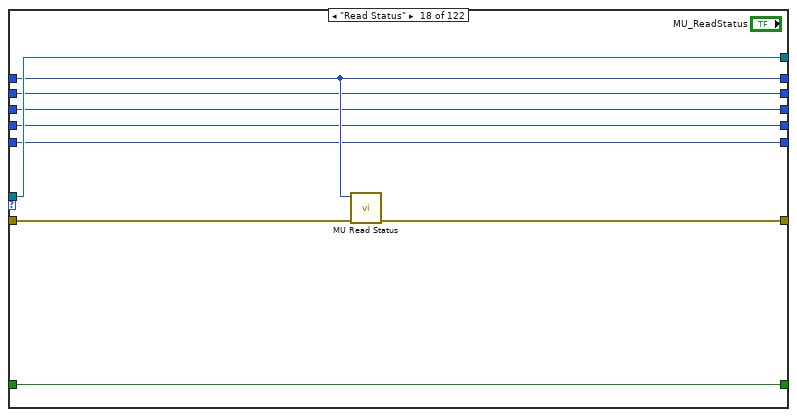
[diagram p19: hidden frame]
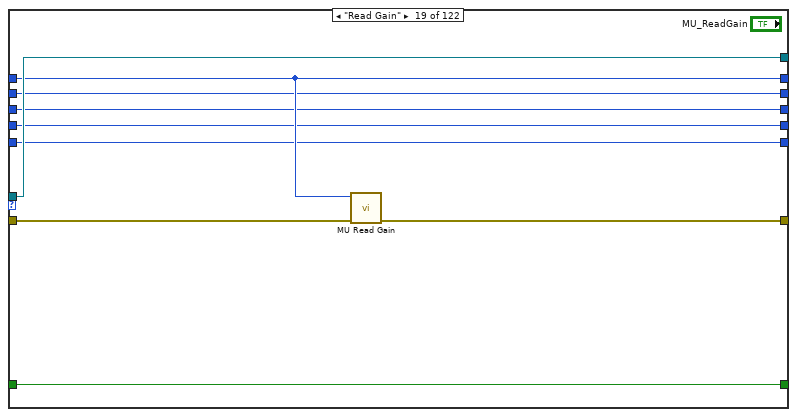
[diagram p20: hidden frame]
diagram:
  w9 = errorcluster {"status"=FALSE, "code"=0, "source"=""}  # error in
  n1 = Obtain Queue(element data type=MU_Functions."Start Demo" ("Events"), error in (no error)=w9) -> (queue out=w12:refnum<queue>, error out=w13:errorcluster)  [unwired: 3 in, 1 out]
  n2 = Enqueue Element(queue=w12, element=MU_Functions."Start Demo" ("Events"), error in (no error)=w13) -> (queue out=w8:refnum<queue>, error out=w7:errorcluster)  [unwired: 1 in, 1 out]
  n3 = while {
    shift-right: [w31] -> _
    shift-left: u64 0 ("pulHTHandle") -> [w30]
    tunnel: [w28] -> _
    shift-right: [w24] -> _
    shift-left: w8 -> [w32]
    tunnel: w7 -> [w23]
    tunnel: FALSE -> [w22]
    shift-right: [w20] -> _
    shift-left: T22 0 ("CalibrationHandle") -> [w21]
    shift-right: [w18] -> _
    shift-left: T21 0 ("CalibrationAnalyzeResultHandle") -> [w19]
    shift-right: [w16] -> _
    shift-left: T20 0 ("mtSyncHandle") -> [w17]
    shift-right: [w15] -> _
    shift-left: T19 0 ("mtSyncAnalyzeResultHandle") -> [w14]
    stop <- w25 stop-if-true
    # "DLL Functions"
    n4 = Dequeue Element(queue=w32, error in (no error)=w23) -> (queue out=w29:refnum<queue>, element=w33:T23, error out=w27:errorcluster)  [unwired: 1 in, 1 out]
    n5 = case shown="\"Calibration_GetOptimizedNoniusTrackOffsetBaseOnly\"" w33 {
      selector: w33 -> [_ _ _ _ _ _ _ _ _ _ _ _ _ _ _ _ _ _ _ _ _ _ _ _ _ _ _ _ _ _ _ _ _ _ _ _ _ _ _ _ _ _ _ _ _ _ _ _ _ _ _ _ _ _ _ _ _ _ _ _ _ _ _ _ _ _ _ _ _ _ _ _ _ _ _ _ _ _ _ _ _ _ _ _ _ _ _ _ _ _ _ _ _ _ _ _ _ _ _ _ _ _ _ _ _ _ _ _ _ _ _ _ _ _ _ _ _ _ _ _ _ w1332]
      tunnel: w27 -> [w39 w52 w61 w72 w82 w93 w104 w113 w124 w137 w146 w153 w167 w178 w189 w200 w209 w216 w225 w237 w247 w258 w268 w275 w284 w290 w303 w313 w323 w333 w343 w353 w363 w373 w382 w393 w403 w414 w427 w435 w445 w455 w465 w475 w491 w500 w509 w521 w533 w545 w557 w562 w574 w594 w606 w616 w626 w636 w645 w654 w664 w674 w684 w694 w704 w714 w724 w734 w745 w755 w765 w778 w788 w798 w807 w818 w827 w836 w847 w857 w866 w875 w884 w893 w904 w913 w926 w939 w955 w966 w977 w987 w998 w1009 w1019 w1027 w1039 w1050 w1065 w1077 w1088 w1098 w1106 w1116 w1126 w1140 w1151 w1163 w1175 w1187 w1193 w1207 w1225 w1236 w1249 w1262 w1275 w1281 w1295 w1311 w1321 w1331]
      tunnel: [w38 w51 w57 w69 w80 w92 w103 w112 w123 w136 w145 w152 w166 w176 w187 w199 w208 w215 w224 w236 w246 w257 w267 w274 w283 w289 w302 w312 w322 w332 w342 w350 w360 w370 w383 w392 w402 w413 w426 w434 w444 w454 w464 w474 w490 w499 w508 w520 w532 w544 w556 w561 w571 w593 w605 w615 w625 w635 w644 w653 w663 w673 w683 w693 w703 w713 w723 w733 w744 w754 w764 w777 w787 w797 w806 w817 w826 w835 w846 w856 w865 w874 w883 w892 w903 w912 w925 w938 w954 w965 w976 w986 w997 w1008 w1018 w1032 w1044 w1055 w1064 w1076 w1087 w1097 w1105 w1115 w1125 w1139 w1150 w1162 w1174 w1186 w1201 w1215 w1224 w1234 w1248 w1261 w1274 w1289 w1303 w1310 w1318 w1330] -> w26
      tunnel: [w41 w48 w58 w67 w77 w87 w98 w114 w125 w134 w143 w154 w160 w173 w184 w196 w205 w217 w226 w233 w243 w254 w264 w276 w285 w296 w309 w319 w329 w339 w349 w359 w369 w379 w389 w399 w410 w421 w432 w442 w452 w462 w472 w482 w492 w501 w510 w522 w534 w546 w558 w569 w580 w595 w607 w617 w627 w637 w646 w655 w665 w675 w685 w695 w705 w715 w725 w735 w746 w756 w766 w779 w789 w799 w808 w819 w828 w837 w848 w858 w867 w876 w885 w894 w905 w914 w927 w940 w956 w967 w978 w988 w999 w1010 w1020 w1029 w1041 w1052 w1066 w1072 w1085 w1095 w1107 w1117 w1127 w1133 w1145 w1159 w1171 w1183 w1198 w1212 w1222 w1232 w1246 w1259 w1272 w1287 w1301 w1312 TRUE w1327] -> w25
      tunnel: [w43 w50 w60 w71 w81 w91 w102 w111 w122 w133 w142 w151 w165 w177 w188 w198 w207 w214 w223 w235 w245 w256 w266 w273 w282 w295 w308 w318 w328 w338 w348 w358 w368 w378 w388 w398 w409 w420 w431 w441 w451 w461 w471 w481 w489 w498 w507 w519 w531 w543 w555 w560 w573 w592 w604 w614 w624 w634 w643 w652 w662 w672 w682 w692 w702 w712 w722 w732 w743 w753 w763 w776 w786 w796 w803 w814 w823 w832 w843 w853 w861 w870 w880 w887 w898 w907 w921 w935 w951 w962 w973 w983 w994 w1005 w1016 w1031 w1043 w1054 w1063 w1075 w1084 w1094 w1104 w1114 w1124 w1138 w1149 w1161 w1173 w1185 w1200 w1214 w1221 w1235 w1245 w1258 w1271 w1286 w1300 w1309 w1319 w1329] -> w31
      tunnel: w30 -> [w43 _ w60 w71 w81 w91 w102 w111 w122 w133 w142 w151 w165 w177 w188 w198 w207 w214 w223 w235 w245 w256 w266 w273 w282 w295 w308 w318 w328 w338 w348 w358 w368 w378 w388 w398 w409 w420 w431 w441 w451 w461 w471 w481 w489 w498 w507 w519 w531 w543 w555 w560 w573 w592 w604 w614 w624 w634 w643 w652 w662 w672 w682 w692 w702 w712 w722 w732 w743 w753 w763 w776 w786 w796 w803 w814 w823 w832 w843 w853 w861 w870 w880 w887 w898 w907 w921 w935 w951 w962 w973 w983 w994 w1005 w1016 w1031 w1043 w1054 w1063 w1075 w1084 w1094 w1104 w1114 w1124 w1138 w1149 w1161 w1173 w1185 w1200 w1214 w1221 w1235 w1245 w1258 w1271 w1286 w1300 w1309 w1319 w1329]
      tunnel: w29 -> [w42 w49 w59 w68 w78 w88 w99 w115 w126 w135 w144 w155 w161 w174 w185 w197 w206 w218 w227 w234 w244 w255 w265 w277 w286 w294 w307 w317 w327 w337 w347 w357 w367 w377 w387 w397 w408 w419 w430 w440 w450 w460 w470 w480 w493 w502 w511 w523 w535 w547 w559 w570 w581 w596 w608 w618 w628 w638 w647 w656 w666 w676 w686 w696 w706 w716 w726 w736 w747 w757 w767 w780 w790 w800 w809 w820 w829 w838 w849 w859 w868 w877 w886 w895 w906 w915 w928 w941 w957 w968 w979 w989 w1000 w1011 w1021 w1030 w1042 w1053 w1067 w1074 w1086 w1096 w1108 w1118 w1128 w1134 w1146 w1160 w1172 w1184 w1199 w1213 w1223 w1233 w1247 w1260 w1273 w1288 w1302 w1313 w1320 w1328]
      tunnel: [w42 w49 w59 w68 w78 w88 w99 w115 w126 w135 w144 w155 w161 w174 w185 w197 w206 w218 w227 w234 w244 w255 w265 w277 w286 w294 w307 w317 w327 w337 w347 w357 w367 w377 w387 w397 w408 w419 w430 w440 w450 w460 w470 w480 w493 w502 w511 w523 w535 w547 w559 w570 w581 w596 w608 w618 w628 w638 w647 w656 w666 w676 w686 w696 w706 w716 w726 w736 w747 w757 w767 w780 w790 w800 w809 w820 w829 w838 w849 w859 w868 w877 w886 w895 w906 w915 w928 w941 w957 w968 w979 w989 w1000 w1011 w1021 w1030 w1042 w1053 w1067 w1074 w1086 w1096 w1108 w1118 w1128 w1134 w1146 w1160 w1172 w1184 w1199 w1213 w1223 w1233 w1247 w1260 w1273 w1288 w1302 w1313 w1320 w1328] -> w24
      tunnel: w22 -> [w41 w48 w58 w67 w77 w87 w98 w114 w125 w134 w143 w154 w160 w173 w184 w196 w205 w217 w226 w233 w243 w254 w264 w276 w285 w296 w309 w319 w329 w339 w349 w359 w369 w379 w389 w399 w410 w421 w432 w442 w452 w462 w472 w482 w492 w501 w510 w522 w534 w546 w558 w569 w580 w595 w607 w617 w627 w637 w646 w655 w665 w675 w685 w695 w705 w715 w725 w735 w746 w756 w766 w779 w789 w799 w808 w819 w828 w837 w848 w858 w867 w876 w885 w894 w905 w914 w927 w940 w956 w967 w978 w988 w999 w1010 w1020 w1029 w1041 w1052 w1066 w1072 w1085 w1095 w1107 w1117 w1127 w1133 w1145 w1159 w1171 w1183 w1198 w1212 w1222 w1232 w1246 w1259 w1272 w1287 w1301 w1312 _ w1327]
      tunnel: w21 -> [w37 w47 w56 w65 w76 w86 w97 w108 w119 w130 w141 w150 w159 w171 w182 w193 w204 w213 w222 w231 w241 w251 w262 _ w281 _ w306 w316 w326 w336 w346 w352 w362 w372 w386 w396 w407 w418 w425 w439 w449 w459 w469 w479 w486 w497 w506 w515 w527 w539 w551 w568 w579 w590 w603 w613 w623 w633 w642 w650 w661 w671 w681 w691 w701 w711 w721 w729 w741 w752 w762 w775 w785 w795 w805 w816 w825 w834 w845 w855 w864 w873 w882 w891 w902 w911 w924 w937 w953 w964 w975 w985 w996 w1007 w1017 w1025 w1036 w1048 w1059 w1071 w1081 w1092 w1102 w1112 w1122 w1132 w1144 w1155 w1167 w1179 w1191 w1205 w1219 w1229 w1240 w1253 w1266 w1279 w1293 w1307 w1317 w1326]
      tunnel: [w37 w47 w56 w65 w76 w86 w97 w108 w119 w130 w141 w150 w159 w171 w182 w193 w204 w213 w222 w231 w241 w251 w262 w272 w281 w288 w306 w316 w326 w336 w346 w352 w362 w372 w386 w396 w407 w418 w425 w439 w449 w459 w469 w479 w486 w497 w506 w515 w527 w539 w551 w568 w579 w590 w603 w613 w623 w633 w642 w650 w661 w671 w681 w691 w701 w711 w721 w729 w741 w752 w762 w775 w785 w795 w805 w816 w825 w834 w845 w855 w864 w873 w882 w891 w902 w911 w924 w937 w953 w964 w975 w985 w996 w1007 w1017 w1025 w1036 w1048 w1059 w1071 w1081 w1092 w1102 w1112 w1122 w1132 w1144 w1155 w1167 w1179 w1191 w1205 w1219 w1229 w1240 w1253 w1266 w1279 w1293 w1307 w1317 w1326] -> w20
      tunnel: w19 -> [w36 w46 w55 w64 w75 w85 w96 w107 w118 w129 w140 w149 w158 w170 w181 w192 w203 w212 w221 w230 w240 w250 w261 w271 w280 w293 w301 w311 w321 w331 w341 w356 w366 w376 w381 w391 w406 w417 w429 w438 w448 w458 w468 w478 w485 w496 w505 w514 w526 w538 w550 w567 w578 w589 _ w611 w622 w632 w641 w651 w660 w670 w680 w690 w700 w710 w720 w731 w742 w750 w760 w774 w784 w794 w804 w815 w824 w833 w844 w854 w863 w872 w881 w890 w901 w910 w923 w933 w952 w963 w974 w984 w995 w1006 w1013 w1024 w1035 w1047 w1058 w1070 w1080 w1091 w1101 w1111 w1121 w1131 w1143 w1154 w1166 w1178 w1190 w1204 w1218 w1228 w1239 w1252 w1265 w1278 w1292 w1306 w1316 w1325]
      tunnel: [w36 w46 w55 w64 w75 w85 w96 w107 w118 w129 w140 w149 w158 w170 w181 w192 w203 w212 w221 w230 w240 w250 w261 w271 w280 w293 w301 w311 w321 w331 w341 w356 w366 w376 w381 w391 w406 w417 w429 w438 w448 w458 w468 w478 w485 w496 w505 w514 w526 w538 w550 w567 w578 w589 w602 w611 w622 w632 w641 w651 w660 w670 w680 w690 w700 w710 w720 w731 w742 w750 w760 w774 w784 w794 w804 w815 w824 w833 w844 w854 w863 w872 w881 w890 w901 w910 w923 w933 w952 w963 w974 w984 w995 w1006 w1013 w1024 w1035 w1047 w1058 w1070 w1080 w1091 w1101 w1111 w1121 w1131 w1143 w1154 w1166 w1178 w1190 w1204 w1218 w1228 w1239 w1252 w1265 w1278 w1292 w1306 w1316 w1325] -> w18
      tunnel: w17 -> [w35 w45 w54 w63 w74 w84 w95 w106 w117 w128 w139 w148 w157 w169 w180 w191 w202 w211 w220 w229 w239 w249 w260 w270 w279 w292 w305 w315 w325 w335 w345 w355 w365 w375 w385 w395 w405 w416 _ w437 w447 w457 w467 w477 w484 w495 w504 w513 w525 w537 w549 w566 w577 w583 w598 w610 w620 w630 w640 w649 w658 w668 w678 w688 w698 w709 w719 w728 w738 w749 w759 w770 w782 w793 w802 w811 w822 _ w840 w851 w862 w871 w878 w888 w899 w908 w922 w936 w949 w961 w972 w982 w993 w1004 w1015 w1023 w1034 w1046 w1057 w1069 w1079 w1090 w1100 w1110 w1120 w1130 w1142 w1153 w1165 w1177 w1189 w1203 w1217 w1227 w1238 w1251 w1264 w1277 w1291 w1305 w1315 w1324]
      tunnel: [w35 w45 w54 w63 w74 w84 w95 w106 w117 w128 w139 w148 w157 w169 w180 w191 w202 w211 w220 w229 w239 w249 w260 w270 w279 w292 w305 w315 w325 w335 w345 w355 w365 w375 w385 w395 w405 w416 w424 w437 w447 w457 w467 w477 w484 w495 w504 w513 w525 w537 w549 w566 w577 w583 w598 w610 w620 w630 w640 w649 w658 w668 w678 w688 w698 w709 w719 w728 w738 w749 w759 w770 w782 w793 w802 w811 w822 w831 w840 w851 w862 w871 w878 w888 w899 w908 w922 w936 w949 w961 w972 w982 w993 w1004 w1015 w1023 w1034 w1046 w1057 w1069 w1079 w1090 w1100 w1110 w1120 w1130 w1142 w1153 w1165 w1177 w1189 w1203 w1217 w1227 w1238 w1251 w1264 w1277 w1291 w1305 w1315 w1324] -> w16
      tunnel: [w34 w44 w53 w62 w73 w83 w94 w105 w116 w127 w138 w147 w156 w168 w179 w190 w201 w210 w219 w228 w238 w248 w259 w269 w278 w291 w304 w314 w324 w334 w344 w354 w364 w374 w384 w394 w404 w415 w428 w436 w446 w456 w466 w476 w483 w494 w503 w512 w524 w536 w548 w565 w576 w582 w597 w609 w619 w629 w639 w648 w657 w667 w677 w687 w697 w708 w718 w727 w737 w748 w758 w769 w781 w792 w801 w810 w821 w830 w839 w850 w860 w869 w879 w889 w900 w909 w920 w934 w950 w960 w971 w981 w992 w1003 w1014 w1022 w1033 w1045 w1056 w1068 w1078 w1089 w1099 w1109 w1119 w1129 w1141 w1152 w1164 w1176 w1188 w1202 w1216 w1226 w1237 w1250 w1263 w1276 w1290 w1304 w1314 w1323] -> w15
      tunnel: w14 -> [w34 w44 w53 w62 w73 w83 w94 w105 w116 w127 w138 w147 w156 w168 w179 w190 w201 w210 w219 w228 w238 w248 w259 w269 w278 w291 w304 w314 w324 w334 w344 w354 w364 w374 w384 w394 w404 w415 w428 w436 w446 w456 w466 w476 w483 w494 w503 w512 w524 w536 w548 w565 w576 w582 w597 w609 w619 w629 w639 w648 w657 w667 w677 w687 w697 w708 w718 w727 w737 w748 w758 w769 w781 w792 w801 w810 w821 w830 _ w850 w860 w869 w879 w889 w900 w909 w920 w934 w950 w960 w971 w981 w992 w1003 w1014 w1022 w1033 w1045 w1056 w1068 w1078 w1089 w1099 w1109 w1119 w1129 w1141 w1152 w1164 w1176 w1188 w1202 w1216 w1226 w1237 w1250 w1263 w1276 w1290 w1304 w1314 w1323]
      frame "Start Demo" {
        n6 = control-ref of="This VI"() -> (w40:refnum<vi>)
        n7 = invoke class="VI" method="Default Vals.Reinit All"(reference=w40, error in=w39) -> (error out=w38:errorcluster)  [unwired: 1 in, 2 out]
      }
      frame "Open" {
        n8 = call "MU Open.vi"("error in (no error)"=w52) -> ("error out (no error)"=w51:errorcluster, "handle"=w50:u64)  [unwired: 8 in, 1 out]
      }
      frame "Close" {
        n9 = call "MU Close.vi"("error in (no error)"=w61, "handle"=w60) -> ("error out (no error)"=w57:errorcluster)  [unwired: 8 in, 1 out]
      }
      frame "Set Interface" {
        n10 = call "MU Set Interface.vi"("error in (no error)"=w72, "interfaceOption"="interfaceOption", "interfaceType"="MU_Interface", "handle"=w71) -> ("error out (no error)"=w69:errorcluster)  [unwired: 6 in, 1 out]
      }
      frame "Get Interface" {
        n11 = call "MU Get Interface.vi"("error in (no error)"=w82, "handle"=w81) -> ("error out (no error)"=w80:errorcluster, "interfaceType"=→"MU_Interface":u32)  [unwired: 7 in, 1 out]
      }
      frame "Set Config" {
        n12 = call "MU Set Config.vi"("error in (no error)"=w93, "value"="value", "configuration"="MU_ConfigData", "handle"=w91) -> ("error out (no error)"=w92:errorcluster)  [unwired: 6 in, 1 out]
      }
      frame "Get Config" {
        n13 = call "MU Get Config.vi"("error in (no error)"=w104, "configuration"="MU_ConfigData", "handle"=w102) -> ("error out (no error)"=w103:errorcluster, "value"=→"value":u32)  [unwired: 6 in, 1 out]
      }
      frame "Switch to BiSS" {
        n14 = call "MU Switch To Biss.vi"("error in (no error)"=w113, "handle"=w111) -> ("error out (no error)"=w112:errorcluster, "modeb"=→"modeb":u32, "modea"=→"modea":u32)  [unwired: 6 in, 1 out]
      }
      frame "Switch to BiSS Ex" {
        n15 = call "MU Switch to BiSS Ex.vi"("error in (no error)"=w124, "handle"=w122) -> ("error out (no error)"=w123:errorcluster, "switched"=→"switched":bool, "modea"=→"modea":u32)  [unwired: 6 in, 1 out]
      }
      frame "Enable Get MT" {
        n16 = call "MU Enable Get MT.vi"("error in (no error)"=w137, "handle"=w133) -> ("error out (no error)"=w136:errorcluster, "switched"=→"switched":bool, "modea"=→"modea":u32)  [unwired: 6 in, 1 out]
      }
      frame "Disable Get MT" {
        n17 = call "MU Disable Get MT.vi"("error in (no error)"=w146, "handle"=w142) -> ("error out (no error)"=w145:errorcluster)  [unwired: 8 in, 1 out]
      }
      frame "Initialize" {
        n18 = call "MU Initialize.vi"("error in (no error)"=w153, "handle"=w151) -> ("error out (no error)"=w152:errorcluster)  [unwired: 8 in, 1 out]
      }
      frame "Set Param" {
        n19 = call "MU Set Param.vi"("writeVerify"="MU_WriteVerifyEnum 2", "error in (no error)"=w167, "value"="ulValue", "parameter"="MU_ParamEnum 3", "handle"=w165) -> ("error out (no error)"=w166:errorcluster)  [unwired: 5 in, 1 out]
      }
      frame "Get Param" {
        n20 = call "MU Get Param.vi"("error in (no error)"=w178, "parameter"="MU_ParamEnum 3", "MUhandle"=w177) -> ("error out (no error)"=w176:errorcluster, "value"=→"pulValue":u64)  [unwired: 6 in, 1 out]
      }
      frame "Is Parameter Available In Used Revision" {
        n21 = call "MU Is Parameter Available In Used Revision.vi"("error in (no error)"=w189, "parameter"="MU_ParamEnum 4", "handle"=w188) -> ("error out (no error)"=w187:errorcluster, "isInRevision"=→"isInRevision":bool)  [unwired: 6 in, 1 out]
      }
      frame "Write Params" {
        n22 = call "MU Write Params.vi"("error in (no error)"=w200, "verify"="verify", "handle"=w198) -> ("error out (no error)"=w199:errorcluster, "valid"=→"valid":bool[])  [unwired: 6 in, 1 out]
      }
      frame "Read Params" {
        n23 = call "MU Read Params.vi"("error in (no error)"=w209, "handle"=w207) -> ("error out (no error)"=w208:errorcluster)  [unwired: 8 in, 1 out]
      }
      frame "Read Status" {
        n24 = call "MU Read Status.vi"("error in (no error)"=w216, "handle"=w214) -> ("error out (no error)"=w215:errorcluster)  [unwired: 8 in, 1 out]
      }
      frame "Read Gain" {
        n25 = call "MU Read Gain.vi"("error in (no error)"=w225, "handle"=w223) -> ("error out (no error)"=w224:errorcluster)  [unwired: 8 in, 1 out]
      }
      frame "Write Eeprom" {
        n26 = call "MU Write Eeprom.vi"("error in (no error)"=w237, "eepromArea"="MU_E2PArea", "handle"=w235) -> ("error out (no error)"=w236:errorcluster)  [unwired: 7 in, 1 out]
      }
      frame "Write Cmd Register" {
        n27 = call "MU Write Cmd Register.vi"("error in (no error)"=w247, "command"="MU_Command", "handle"=w245) -> ("error out (no error)"=w246:errorcluster)  [unwired: 7 in, 1 out]
      }
      frame "Write Switch Command" {
        n28 = call "MU Write Switch Command.vi"("error in (no error)"=w258, "rplNew"="rplNew", "modeaNew"="modeaNew", "handle"=w256) -> ("error out (no error)"=w257:errorcluster)  [unwired: 6 in, 1 out]
      }
      frame "Read Sens" {
        n29 = call "MU Read Sens.vi"("error in (no error)"=w268, "handle"=w266) -> ("error out (no error)"=w267:errorcluster, "data"=→"data":T9)  [unwired: 7 in, 1 out]
      }
      frame "Get Calibration" {
        n30 = call "MU get Calibration.vi"("error in (no error)"=w275, "MUhandle"=w273) -> ("error out"=w274:errorcluster, "CalibrationHandle"=w272:T22)  [unwired: 8 in]
      }
      frame "Set Calibration" {
        n31 = call "MU set Calibration.vi"("error in (no error)"=w284, "CalibrationHandle"=w281, "MUhandle"=w282) -> ("error out"=w283:errorcluster)  [unwired: 7 in, 1 out]
      }
      frame "Calibration_createCalibration" {
        n32 = call "MU create Calibration.vi"("error in (no error)"=w290, "revisionCode"="revisionCode") -> ("error out"=w289:errorcluster, "CalibrationHandle"=w288:T22)  [unwired: 8 in]
      }
      frame "Calibration_getAnalyzeResultLog" {
        n33 = call "MU Calibration Get Analyze Result Log.vi"("error in (no error)"=w303, "logLevel"="MU_AdjustmentLogLevel", "logDestSize"="logDestSize", "analyzeResult"=w301) -> ("error out (no error)"=w302:errorcluster, "logDest"=→"logDest":string, "size"=→"size":u64)  [unwired: 5 in]
      }
      frame "Calibration_minimalNumberOfSamplesPerMasterPeriod" {
        n34 = call "MU Calibration Minimal Number Of Samples Per Master Period.vi"("error in (no error)"=w313, "AnalyzeResultHandle"=w311) -> ("error out (no error)"=w312:errorcluster, "minimalNumberOfSamplesPerMasterPeriod"=→"minimalNumberOfSamplesPerMasterPeriod":dbl)  [unwired: 8 in]
      }
      frame "Calibration_noniusPhaseRangeLimit" {
        n35 = call "MU Calibration Nonius Phase Range Limit.vi"("error in (no error)"=w323, "AnalyzeResultHandle"=w321) -> ("error out"=w322:errorcluster, "NoniusPhaseRangeLimit"=→"noniusPhaseRangeLimit":i32)  [unwired: 8 in]
      }
      frame "Calibration_noniusUpperPhaseMargin" {
        n36 = call "MU Calibration Nonius Upper Phase Margin.vi"("error in (no error)"=w333, "AnalyzeResultHandle"=w331) -> ("error out"=w332:errorcluster, "NoniusUpperPhaseMargin"=→"noniusUpperPhaseMargin":dbl)  [unwired: 8 in]
      }
      frame "Calibration_noniusLowerPhaseMargin" {
        n37 = call "MU Calibration Nonius Lower Phase Margin.vi"("error in (no error)"=w343, "AnalyzeResultHandle"=w341) -> ("error out"=w342:errorcluster, "NoniusLowerPhaseMargin"=→"noniusLowerPhaseMargin":dbl)  [unwired: 8 in]
      }
      frame "Calibration_getAnalogMasterTrackAdjustments" {
        n38 = call "MU Calibration Get Analog Master Track Adjustments.vi"("error in (no error)"=w353, "CalibrationHandle"=w352) -> ("error out"=w350:errorcluster, "masterAdjustments"=→"masterAdjustments":T13)  [unwired: 8 in]
      }
      frame "Calibration_getAnalogNoniusTrackAdjustments" {
        n39 = call "MU Calibration Get Analog Nonius Track Adjustments.vi"("error in (no error)"=w363, "CalibrationHandle"=w362) -> ("error out"=w360:errorcluster, "noniusAdjustments"=→"noniusAdjustments":T13)  [unwired: 8 in]
      }
      frame "Calibration_getNoniusTrackOffsetTable" {
        n40 = call "MU Calibration Get Nonius Track Offset Table.vi"("error in (no error)"=w373, "CalibrationHandle"=w372) -> ("error out (no error)"=w370:errorcluster, "noniusTrackOffsetTable"=→"NoniusTrackOffsetTable":cluster{"spoBase":i8, "spoN":i8[]})  [unwired: 8 in]
      }
      frame "Calibration_isAnalogAnalysesValid" {
        n41 = call "MU Calibration Is Analog Analyses Valid.vi"("error in (no error)"=w382, "AnalyzeResultHandle"=w381) -> ("error out"=w383:errorcluster, "isAnalogAnalysesValid"=→"isAnalogAnalysesValid":bool)  [unwired: 8 in]
      }
      frame "Calibration_isNoniusAnalysesValid" {
        n42 = call "MU Calibration Is Nonius Analyses Valid.vi"("error in (no error)"=w393, "AnalyzeResultHandle"=w391) -> ("error out"=w392:errorcluster, "isNoniusAnalysesValid"=→"isNoniusAnalysesValid":bool)  [unwired: 8 in]
      }
      frame "getNoniusTrackOffsetTableParameters" {
        n43 = call "MU Get Nonius Track Offset Table Parameters.vi"("error in (no error)"=w403, "noniusTrackOffsetTable"="noniusTrackOffsetTable") -> ("error out (no error)"=w402:errorcluster, "noniusTrackOffsetTableParameters"=→"noniusTrackOffsetTableParameters":cluster{"spoBase":u8, "spoN":u8[]})  [unwired: 8 in]
      }
      frame "getNoniusTrackOffsetTableByParameters" {
        n44 = call "MU Get Nonius Track Offset Table By Parameters.vi"("error in (no error)"=w414, "noniusTrackOffsetTableParameters"="noniusTrackOffsetTableParameters") -> ("error out (no error)"=w413:errorcluster, "noniusTrackOffsetTable"=→"noniusTrackOffsetTable":cluster{"spoBase":i8, "spoN":i8[]})  [unwired: 8 in]
      }
      frame "createMtSync" {
        n45 = call "MU Create Mt Sync.vi"("error in (no error)"=w427, "mtMovementIsReverse"="mtMovementIsReverse", "nMtSyncBits"="nMtSyncBits", "CalibrationHandle"=w425) -> ("error out"=w426:errorcluster, "mtSyncHandle"=w424:T20)  [unwired: 6 in]
      }
      frame "getVersionMajor" {
        n46 = call "MU Get Version Major.vi"("error in (no error)"=w435) -> ("error out (no error)"=w434:errorcluster, "versionMajor"=→"versionMajor":u16)  [unwired: 9 in]
      }
      frame "getVersionMinor" {
        n47 = call "MU Get Version Minor.vi"("error in (no error)"=w445) -> ("error out (no error)"=w444:errorcluster, "versionMinor"=→"versionMinor":u16)  [unwired: 9 in]
      }
      frame "getVersionPatch" {
        n48 = call "MU Get Version Patch.vi"("error in (no error)"=w455) -> ("error out (no error)"=w454:errorcluster, "versionPatch"=→"versionPatch":u16)  [unwired: 9 in]
      }
      frame "getVersionBuild" {
        n49 = call "MU Get Version Build.vi"("error in (no error)"=w465) -> ("error out (no error)"=w464:errorcluster, "versionBuild"=→"versionBuild":u16)  [unwired: 9 in]
      }
      frame "getVersionSuffixString" {
        n50 = call "MU Get Version Suffix String.vi"("error in (no error)"=w475) -> ("error out (no error)"=w474:errorcluster, "versionSuffixString"=→"versionSuffixString":string)  [unwired: 9 in]
      }
      frame "Calibration_setCurrentAnalogTrackAdjustments" {
        n51 = call "MU Calibration set Current Analog Track Adjustments.vi"("error in (no error)"=w491, "noniusAdjustments"="noniusAdjustments", "masterAdjustments"="masterAdjustments", "CalibrationHandle"=w486) -> ("error out"=w490:errorcluster)  [unwired: 6 in, 1 out]
      }
      frame "ActivateCalibrationConfig" {
        n52 = call "MU Activate Calibration Config.vi"("error in (no error)"=w500, "MUhandle"=w498) -> ("error out"=w499:errorcluster)  [unwired: 8 in, 1 out]
      }
      frame "DeactivateCalibrationConfig" {
        n53 = call "MU Deactivate Calibration Config.vi"("error in (no error)"=w509, "MUhandle"=w507) -> ("error out"=w508:errorcluster)  [unwired: 8 in, 1 out]
      }
      frame "InterfaceNearestPossibleClockFreq" {
        n54 = call "MU Interface Nearest Possible Clock Freq.vi"("error in (no error)"=w521, "clockFrequency_hz"="clockFrequency_hz", "interfaceType"="MU_Interface") -> ("error out (no error)"=w520:errorcluster, "nearestClockFrequency"=→"nearestClockFrequency":dbl)  [unwired: 7 in]
      }
      frame "InterfaceNearestPossibleFrameCycleTime" {
        n55 = call "MU Interface Nearest Possible Frame Cycle Time.vi"("error in (no error)"=w533, "frameCycleTime_s"="frameCycleTime_s", "interfaceType"="MU_Interface") -> ("error out (no error)"=w532:errorcluster, "nearestFrameCycleTime"=→"nearestFrameCycleTime":dbl)  [unwired: 7 in]
      }
      frame "InterfaceNextPossibleFrameCycleTime" {
        n56 = call "MU Interface Next Possible Frame Cycle Time.vi"("error in (no error)"=w545, "frameCycleTime_s"="frameCycleTime_s", "interfaceType"="MU_Interface") -> ("error out (no error)"=w544:errorcluster, "nextFrameCycleTime"=→"nextFrameCycleTime":dbl)  [unwired: 7 in]
      }
      frame "InterfaceNextPossibleClockFreq" {
        n57 = call "MU Interface Next Possible Clock Freq.vi"("error in (no error)"=w557, "clockFrequency_hz"="clockFrequency_hz", "interfaceType"="MU_Interface") -> ("error out (no error)"=w556:errorcluster, "nextClockFrequency"=→"nextClockFrequency":dbl)  [unwired: 7 in]
      }
      frame "generateBissIdentifier" {
        n58 = call "MU generate Biss Identifier.vi"("Error In"=w562, "handle"=w560) -> ("Error Out"=w561:errorcluster, "mfgID"=→"mfgID":u16, "deviceID"=→"deviceID":u64)  [unwired: 6 in, 1 out]
      }
      frame "generateBissProfileId" {
        n59 = call "MU generate Biss Profile Id.vi"("Error In"=w574, "profile"="MU_BissProfile", "handle"=w573) -> ("Error Out"=w571:errorcluster, "bissProfileId"=→"bissProfileId":u16)  [unwired: 6 in, 1 out]
      }
      frame "AcquireRawData" {
        n60 = call "MU acquire Raw Data.vi"("clockFrequency"="clockFrequency", "frameCycleTime"="frameCycleTime", "error in (no error)"=w594, "SlaveID"="SlaveID", "numberOfSamples"="numberOfSamples", "MUhandle"=w592) -> ("error out"=w593:errorcluster, "noniusRawData"=→"noniusRawData":u16[], "masterRawData"=→"masterRawData":u16[])  [unwired: 2 in, 1 out]
      }
      frame "Calibration_AnalyzeRawData" {
        n61 = call "MU Calibration analyze Raw Data.vi"("numberOfRawDataSamples"="numberOfRawDataSamples", "error in (no error)"=w606, "noniusTrackRawData"="noniusTrackRawData", "masterTrackRawData"="masterTrackRawData", "CalibrationHandle"=w603) -> ("error out (no error)"=w605:errorcluster, "CalibrationAnalyzeResultHandle"=w602:T21)  [unwired: 5 in]
      }
      frame "Calibration_GetRelativeMasterTrackAdjustments" {
        n62 = call "MU Calibration Get Relative Master Track Adjustments.vi"("error in (no error)"=w616, "CalibrationAnalyzeResult"=w611) -> ("error out (no error)"=w615:errorcluster, "MU_Calibration_RelativeAnalogTrackAdjustments_Master"=→"MU_Calibration_RelativeAnalogTrackAdjustments_Master":T11)  [unwired: 8 in]
      }
      frame "Calibration_GetRelativeNoniusTrackAdjustment" {
        n63 = call "MU Calibration Get Relative Nonius Track Adjustments.vi"("error in (no error)"=w626, "CalibrationAnalyzeResult"=w622) -> ("error out (no error)"=w625:errorcluster, "MU_Calibration_RelativeAnalogTrackAdjustments_Nonius"=→"MU_Calibration_RelativeAnalogTrackAdjustments_Nonius":T11)  [unwired: 8 in]
      }
      frame "Calibration_AdjustAnalogByAnalyzeResult" {
        n64 = call "MU Calibration adjust Analog By Analyze Result.vi"("error in (no error)"=w636, "analyzeResult"=w632, "calibration"=w633) -> ("error out"=w635:errorcluster, "function return"=→"function return":bool)  [unwired: 7 in]
      }
      frame "Calibration_AnalyzeResultdelete" {
        n65 = call "MU Calibration delete Analyze Result.vi"("error in (no error)"=w645, "analyzeResult"=w641) -> ("error out"=w644:errorcluster)  [unwired: 9 in]
      }
      frame "Calibration_delete" {
        n66 = call "MU Calibration delete.vi"("error in (no error)"=w654, "calibration"=w650) -> ("error out"=w653:errorcluster)  [unwired: 9 in]
      }
      frame "Calibration_NumberOfCalculatedMasterPeriods" {
        n67 = call "MU Calibration Number Of Calculated Master Periods.vi"("error in (no error)"=w664, "analyzeResult"=w660) -> ("error out (no error)"=w663:errorcluster, "CalculatedMasterPeriods"=→"CalculatedMasterPeriods":i32)  [unwired: 8 in]
      }
      frame "Calibration_NumberOfNoniusCurveSamples" {
        n68 = call "MU Calibration Number Of Nonius Curve Samples.vi"("error in (no error)"=w674, "CalibrationAnalyzeResult"=w670) -> ("error out"=w673:errorcluster, "NumberOfNoniusCurveSamples"=→"NumberOfNoniusCurveSamples":u64)  [unwired: 8 in]
      }
      frame "Calibration_NoniusPhaseError" {
        n69 = call "MU Calibration Nonius Phase Error.vi"("error in (no error)"=w684, "analyzeResult"=w680) -> ("error out"=w683:errorcluster, "PhaseError"=→"PhaseError":i32[])  [unwired: 7 in, 1 out]
      }
      frame "Calibration_NoniusTrackOffsetCurve" {
        n70 = call "MU Calibration Nonius Track Offset Curve.vi"("error in (no error)"=w694, "analyzeResult"=w690) -> ("error out"=w693:errorcluster, "TrackOffset"=→"TrackOffset":i32[])  [unwired: 7 in, 1 out]
      }
      frame "Calibration_NoniusPhaseMargin" {
        n71 = call "MU Calibration Nonius Phase Margin.vi"("error in (no error)"=w704, "analyzeResult"=w700) -> ("error out"=w703:errorcluster, "PhaseMargin"=→"PhaseMargin":i32[])  [unwired: 7 in, 1 out]
      }
      frame "Calibration_GetOptimizedNoniusTrackOffsetTable" {
        n72 = call "MU Calibration Get Optimized Nonius Track Offset Table.vi"("error in (no error)"=w714, "analyzeResult"=w710) -> ("error out (no error)"=w713:errorcluster, "optimizedNoniusTrackOffsetTable"=→"optimizedNoniusTrackOffsetTable":cluster{"spoBase":i8, "spoN":i8[]})  [unwired: 8 in]
      }
      frame "Calibration_GetOptimizedNoniusTrackOffsetBaseOnly" {
        n73 = call "MU Calibration Get Optimized Nonius Track Offset Table Base Only.vi"("error in (no error)"=w724, "analyzeResult"=w720) -> ("error out (no error)"=w723:errorcluster, "optimizedNoniusTrackOffsetTableBaseOnly"=→"optimizedNoniusTrackOffsetTableBaseOnly":cluster{"spoBase":i8, "spoN":i8[]})  [unwired: 8 in]
      }
      frame "Calibration_SetCurrentNoniusTrackOffsetTable" {
        n74 = call "MU Calibration Set Current Nonius Track Offset Table.vi"("error in (no error)"=w734, "optimizedNoniusTrackOffsetTable"="optimizedNoniusTrackOffsetTable", "CalibrationHandle"=w729) -> ("error out (no error)"=w733:errorcluster)  [unwired: 7 in, 1 out]
      }
      frame "Calibration_PreconfigureNumberOfMasterPeriods" {
        n75 = call "MU Calibration Preconfigure Number Of Master Periods.vi"("error in (no error)"=w745, "NumberOfMasterPeriods (0=autodetect)"="NumberOfMasterPeriods (0=autodetect)", "calibration"=w741) -> ("error out"=w744:errorcluster, "Return value"=→"Return value":bool)  [unwired: 7 in]
      }
      frame "Calibration_NoniusPhaseMarginMax" {
        n76 = call "MU Calibration Nonius Phase Margin Max.vi"("error in (no error)"=w755, "AnalyzeResultHandle"=w750) -> ("error out"=w754:errorcluster, "NoniusPhaseMarginMax"=→"NoniusPhaseMarginMax":i32)  [unwired: 8 in]
      }
      frame "Calibration_NoniusPhaseMarginMin" {
        n77 = call "MU Calibration Nonius Phase Margin Min.vi"("error in (no error)"=w765, "AnalyzeResultHandle"=w760) -> ("error out"=w764:errorcluster, "NoniusPhaseMarginMin"=→"NoniusPhaseMarginMin":i32)  [unwired: 8 in]
      }
      frame "Calibration_IsAnalogAnalyzeResultAdjustable" {
        n78 = call "MU Calibration Is Analog Analyze Result Adjustable.vi"("adjustmentMessageLogLevel"="MU_AdjustmentLogLevel", "error in (no error)"=w778, "adjustmentMessageBufferSize"="adjustmentMessageBufferSize", "analyzeResult"=w774, "CalibrationHandle"=w775) -> ("error out (no error)"=w777:errorcluster, "adjustMessage"=→"adjustMessage":string, "Result"=→"Result":bool)  [unwired: 4 in]
      }
      frame "Calibration_NumberOfAcquiredMasterPeriods" {
        n79 = call "MU Calibration Number Of Acquired Master Periods.vi"("error in (no error)"=w788, "analyzeResult"=w784) -> ("error out (no error)"=w787:errorcluster, "AcquiredPeriods"=→"acquiredMasterPeriods":dbl)  [unwired: 8 in]
      }
      frame "Calibration_NumberOfAcquiredNoniusPeriods" {
        n80 = call "MU Calibration Number Of Acquired Nonius Periods.vi"("error in (no error)"=w798, "analyzeResult"=w794) -> ("error out (no error)"=w797:errorcluster, "AcquiredPeriods"=→"acquiredNoniusPeriods":dbl)  [unwired: 8 in]
      }
      frame "ActivateMtSyncConfig" {
        n81 = call "MU Activate Mt Sync Config.vi"("error in (no error)"=w807, "MUhandle"=w803) -> ("error out"=w806:errorcluster)  [unwired: 8 in, 1 out]
      }
      frame "AcquireMtSyncData" {
        n82 = call "MU Acquire MtSync Data.vi"("error in (no error)"=w818, "numberOfSamples"="Samples", "MUhandle"=w814) -> ("error out (no error)"=w817:errorcluster, "data"=→"data":T15)  [unwired: 6 in, 1 out]
      }
      frame "DeactivateMtSyncConfig" {
        n83 = call "MU Deactivate Mt Sync Config.vi"("error in (no error)"=w827, "MUhandle"=w823) -> ("error out"=w826:errorcluster)  [unwired: 8 in, 1 out]
      }
      frame "GetMtSync" {
        n84 = call "MU Get Mt Sync.vi"("error in (no error)"=w836, "MUhandle"=w832) -> ("error out"=w835:errorcluster, "mtSyncHandle"=w831:T20)  [unwired: 8 in]
      }
      frame "MtSync_analyzeData" {
        n85 = call "MU Mt Sync Analyze Data.vi"("error in (no error)"=w847, "numberOfSamples"="numberOfSamples", "data"="data", "mtSyncHandle"=w840) -> ("error out"=w846:errorcluster, "mtSyncAnalyzeResultHandle"=w839:T19)  [unwired: 6 in]
      }
      frame "MtAnalyzeResult_optimalSpoMt" {
        n86 = call "MU Mt Analyze Result Optimal Spo_Mt.vi"("error in (no error)"=w857, "mtSyncAnalyzeResultHandle"=w850) -> ("error out"=w856:errorcluster, "optimalSpoMt"=→"optimalSpoMt":u8)  [unwired: 8 in]
      }
      frame "UpdateMtSync" {
        n87 = call "MU Update Mt Sync.vi"("error in (no error)"=w866, "MtAnalyzeResultHandle"=w860, "MuHandle"=w861) -> ("error out"=w865:errorcluster)  [unwired: 7 in, 1 out]
      }
      frame "MtAnalyzeResult_delete" {
        n88 = call "MU Mt Analyze Result Delete.vi"("error in (no error)"=w875, "mtSynchAnalyzeResultHandle"=w869) -> ("error out"=w874:errorcluster)  [unwired: 9 in]
      }
      frame "MtSync_delete" {
        n89 = call "MU Mt Sync Delete.vi"("error in (no error)"=w884, "mtSyncHandle"=w878) -> ("error out"=w883:errorcluster)  [unwired: 9 in]
      }
      frame "Activate3TrackMtSyncConfig" {
        n90 = call "MU Activate 3 Track Mt Sync Config.vi"("error in (no error)"=w893, "MUhandle"=w887) -> ("error out"=w892:errorcluster)  [unwired: 8 in, 1 out]
      }
      frame "Acquire3TrackMtSyncData" {
        n91 = call "MU Acquire 3 Track Mt Sync Data.vi"("error in (no error)"=w904, "Samples"="Samples", "MUhandle"=w898) -> ("error out"=w903:errorcluster, "SyncData"=→"SyncData":T14)  [unwired: 6 in, 1 out]
      }
      frame "Deactivate3TrackMtSyncConfig" {
        n92 = call "MU Deactivate 3 Track Mt Sync Config.vi"("error in (no error)"=w913, "MUhandle"=w907) -> ("error out"=w912:errorcluster)  [unwired: 8 in, 1 out]
      }
      frame "MtAnalyzeResult_calculateOffsetError" {
        n93 = call "MU Mt Analyze Result Calculate Offset Error.vi"("error in (no error)"=w926, "MtTrackOffset"="MtTrackOffset", "Samples"="Samples", "MtSync_AnalyzeResultHandle"=w920) -> ("error out"=w925:errorcluster, "MT_OffsetError"=→"MT_OffsetError":dbl[], "Return Value"=→"Return Value":u64)  [unwired: 5 in]
      }
      frame "Calibration_calculateNoniusPosition" {
        n94 = call "MU Calibration Calculate Nonius Position.vi"("error in (no error)"=w939, "Continuous"="Continuous", "Calibration Unit"="MU_Unit", "analyzeResult"=w933) -> ("error out"=w938:errorcluster, "SingleturnPosition"=→"SingleturnPosition":dbl[], "Return Value"=→"Return Value":u64)  [unwired: 5 in]
      }
      frame "MtSync_calculatePosition" {
        n95 = call "MU Mt Sync Calculate Position.vi"("Continuous (F)"="Continuous (F)", "Calibration Unit"="Calibration Unit", "resolution"="resolution", "MtTrackOffset"="MtTrackOffset", "error in (no error)"=w955, "Samples"="Samples", "SyncData"="SyncData", "mtSyncHandle"=w949) -> ("error out"=w954:errorcluster, "MT_Position"=→"MT_Position":dbl[])  [unwired: 1 in, 1 out]
      }
      frame "MtAnalyzeResult_maxOffsetError" {
        n96 = call "MU Mt Analyze Result Max Offset Error.vi"("error in (no error)"=w966, "MtTrackOffset"="MtTrackOffset", "MtSync_AnalyzeResultHandle"=w960) -> ("error out"=w965:errorcluster, "MaxOffsetError"=→"MaxOffsetError":dbl)  [unwired: 7 in]
      }
      frame "MtAnalyzeResult_minOffsetError" {
        n97 = call "MU Mt Analyze Result Min Offset Error.vi"("error in (no error)"=w977, "MtTrackOffset"="MtTrackOffset", "MtSync_AnalyzeResultHandle"=w971) -> ("error out"=w976:errorcluster, "MinOffsetError"=→"MinOffsetError":dbl)  [unwired: 7 in]
      }
      frame "MtAnalyzeResult_offsetErrorRangeLimit" {
        n98 = call "MU Mt Analyze Result Offset Error Range Limit.vi"("error in (no error)"=w987, "MtSync_AnalyzeResultHandle"=w981) -> ("error out"=w986:errorcluster, "OffsetErrorRangeLimit"=→"OffsetErrorRangeLimit":dbl)  [unwired: 8 in]
      }
      frame "MtAnalyzeResult_lowerOffsetErrorMargin" {
        n99 = call "MU Mt Analyze Result Lower Offset Error Margin.vi"("error in (no error)"=w998, "MtTrackOffset"="MtTrackOffset", "MtSync_AnalyzeResultHandle"=w992) -> ("error out"=w997:errorcluster, "LowerOffsetErrorMargin"=→"LowerOffsetErrorMargin":dbl)  [unwired: 7 in]
      }
      frame "MtAnalyzeResult_upperOffsetErrorMargin" {
        n100 = call "MU Mt Analyze Result Upper Offset Error Margin.vi"("error in (no error)"=w1009, "MtTrackOffset"="MtTrackOffset", "analyzeResultHandle"=w1003) -> ("error out"=w1008:errorcluster, "UpperOffsetErrorMargin"=→"UpperOffsetErrorMargin":dbl)  [unwired: 7 in]
      }
      frame "Calibration_numberOfRevolutions" {
        n101 = call "MU Calibration Number Of Revolutions.vi"("error in (no error)"=w1019, "AnalyzeResultHandle"=w1013) -> ("error out (no error)"=w1018:errorcluster, "NumberOfRevolutions"=→"NumberOfRevolutions":dbl)  [unwired: 8 in]
      }
      frame "Save Params" {
        n102 = Path To String(path="pcCfgFilename") -> (string=w1028:string)
        n103 = call "MU Save Params.vi"("error in (no error)"=w1027, "filepath"=w1028, "handle"=w1031) -> ("error out (no error)"=w1032:errorcluster)  [unwired: 7 in, 1 out]
      }
      frame "Read Chip Revision Of Parameter File" {
        n104 = Path To String(path="pcCfgFilename 5") -> (string=w1040:string)
        n105 = call "MU Read Chip Revision Of Parameter File.vi"("error in (no error)"=w1039, "filepath"=w1040, "handle"=w1043) -> ("error out (no error)"=w1044:errorcluster, "revisionCode"=→"revisionCode":u32)  [unwired: 6 in, 1 out]
      }
      frame "Load Params" {
        n106 = Path To String(path="pcCfgFilename 2") -> (string=w1051:string)
        n107 = call "MU Load Params.vi"("error in (no error)"=w1050, "filepath"=w1051, "handle"=w1054) -> ("error out (no error)"=w1055:errorcluster)  [unwired: 7 in, 1 out]
      }
      frame "Get Last Error" {
        n108 = call "MU Get Last Error.vi"("error in (no error)"=w1065, "handle"=w1063) -> ("error out (no error)"=w1064:errorcluster, "lastErrorType"=→"MU_ErrorType":u32, "lastError"=→"MU_Error":u32, "lastErrorText"=→"lastErrorText":string)  [unwired: 5 in, 1 out]
      }
      frame "Get DLL Version" {
        n109 = call "MU Get DLL Version.vi"("error in (no error)"=w1077) -> ("error out (no error)"=w1076:errorcluster, "version"=→"version":u32[])  [unwired: 8 in, 1 out]
      }
      frame "Calc PRES_POS" {
        n110 = call "MU Calc PRES_POS.vi"("writeVerify"="MU_WriteVerifyEnum", "error in (no error)"=w1088, "value"="value", "handle"=w1084) -> ("error out (no error)"=w1087:errorcluster)  [unwired: 7 in]
      }
      frame "Get PRES_POS" {
        n111 = call "MU Get PRES_POS.vi"("error in (no error)"=w1098, "handle"=w1094) -> ("error out (no error)"=w1097:errorcluster, "value"=→"value":u64)  [unwired: 7 in, 1 out]
      }
      frame "Use Revision" {
        n112 = call "MU Use Revision.vi"("error in (no error)"=w1106, "revisionId"="revisionId", "handle"=w1104) -> ("error out (no error)"=w1105:errorcluster)  [unwired: 7 in, 1 out]
      }
      frame "Value Of Used Revision" {
        n113 = call "MU Value Of Used Revision.vi"("error in (no error)"=w1116, "handle"=w1114) -> ("error out (no error)"=w1115:errorcluster, "revisionId"=→"revisionId":u32)  [unwired: 7 in, 1 out]
      }
      frame "Read Chip Revision" {
        n114 = call "MU Read Chip Revision.vi"("error in (no error)"=w1126, "handle"=w1124) -> ("error out (no error)"=w1125:errorcluster, "revisionId"=→"revisionId":u32)  [unwired: 7 in, 1 out]
      }
      frame "Set Register" {
        n115 = call "MU Set Register.vi"("writeVerify"="MU_WriteVerifyEnum 2", "error in (no error)"=w1140, "value"="ulValue", "address"="address", "handle"=w1138) -> ("error out (no error)"=w1139:errorcluster)  [unwired: 5 in, 1 out]
      }
      frame "Get Register" {
        n116 = call "MU Get Register.vi"("error in (no error)"=w1151, "address"="ulAdr", "handle"=w1149) -> ("error out (no error)"=w1150:errorcluster, "value"=→"pulValue":u32)  [unwired: 6 in, 1 out]
      }
      frame "Write Register" {
        n117 = call "MU Write Register.vi"("values"="values", "error in (no error)"=w1163, "count in"="count", "address"="address", "handle"=w1161) -> ("error out (no error)"=w1162:errorcluster)  [unwired: 4 in, 2 out]
      }
      frame "Read Register" {
        n118 = call "MU Read Register.vi"("error in (no error)"=w1175, "count in"="count", "address"="address", "handle"=w1173) -> ("error out (no error)"=w1174:errorcluster, "values"=→"values":u32[])  [unwired: 4 in, 2 out]
      }
      frame "Write Register SSI" {
        n119 = call "MU Write Register SSI.vi"("values"="values", "error in (no error)"=w1187, "count in"="count", "address"="address", "handle"=w1185) -> ("error out (no error)"=w1186:errorcluster)  [unwired: 4 in, 2 out]
      }
      frame "Save Register" {
        n120 = Path To String(path="pcFilename") -> (string=w1197:string)
        n121 = call "MU Save Register.vi"("values"="values", "count in"="count", "error in (no error)"=w1193, "address"="address", "filepath"=w1197, "handle"=w1200) -> ("error out (no error)"=w1201:errorcluster)  [unwired: 3 in, 2 out]
      }
      frame "Load Register" {
        n122 = Path To String(path="pcCfgFilename 3") -> (string=w1211:string)
        n123 = call "MU Load Register.vi"("count in"="count", "error in (no error)"=w1207, "address"="address", "filepath"=w1211, "handle"=w1214) -> ("error out (no error)"=w1215:errorcluster, "values"=→"values":u32[])  [unwired: 3 in, 2 out]
      }
      frame "Spi Activate" {
        n124 = call "MU Spi Activate.vi"("error in (no error)"=w1225, "data"="data", "handle"=w1221) -> ("error out (no error)"=w1224:errorcluster)  [unwired: 7 in, 1 out]
      }
      frame "Get Interface Info" {
        n125 = call "MU Get Interface Info.vi"("error in (no error)"=w1236, "informationType"="MU_InterfaceInfo", "handle"=w1235) -> ("error out (no error)"=w1234:errorcluster, "information"=→"information":string)  [unwired: 6 in, 1 out]
      }
      frame "Write Register I2C" {
        n126 = call "MU Write Register I2C.vi"("values"="values", "i2cSlaveAddress"="i2cSlaveAddress", "error in (no error)"=w1249, "registerCount"="registerCount", "registerAddress"="registerAddress", "handle"=w1245) -> ("error out (no error)"=w1248:errorcluster)  [unwired: 4 in, 1 out]
      }
      frame "Write Register I2C Ex" {
        n127 = call "MU Write Register I2C Ex.vi"("valid"="valid", "values"="values", "error in (no error)"=w1262, "i2cSlaveAddress"="i2cSlaveAddress", "registerCount"="registerCount", "handle"=w1258) -> ("error out (no error)"=w1261:errorcluster)  [unwired: 4 in, 1 out]
      }
      frame "Read Register I2C" {
        n128 = call "MU Read Register I2C.vi"("i2cSlaveAddress"="i2cSlaveAddress", "error in (no error)"=w1275, "registerCount"="registerCount", "registerAddress"="registerAddress", "handle"=w1271) -> ("error out (no error)"=w1274:errorcluster, "values"=→"values":u32[])  [unwired: 3 in, 2 out]
      }
      frame "Save Register Ex" {
        n129 = Path To String(path="pcFilename 2") -> (string=w1285:string)
        n130 = call "MU Save Register Ex.vi"("values"="values", "registerCount"="registerCount", "error in (no error)"=w1281, "registerAddress"="registerAddress", "filepath"=w1285, "handle"=w1286) -> ("error out (no error)"=w1289:errorcluster)  [unwired: 4 in, 1 out]
      }
      frame "Load Register Ex" {
        n131 = Path To String(path="pcCfgFilename 4") -> (string=w1299:string)
        n132 = call "MU Load Register Ex.vi"("error in (no error)"=w1295, "registerCount"="registerCount", "filepath"=w1299, "handle"=w1300) -> ("error out (no error)"=w1303:errorcluster, "valid"=→"valid":bool[], "values"=→"values":u32[])  [unwired: 4 in, 1 out]
      }
      frame "Get Version String" {
        n133 = call "MU Get Version String.vi"("error in (no error)"=w1311) -> ("error out (no error)"=w1310:errorcluster, "versionString"=→"versionString":string)  [unwired: 9 in]
      }
      frame "Stop Demo" {
        n134 = Release Queue(queue=w1320, error in (no error)=w1321) -> (error out=w1318:errorcluster)  [unwired: 1 in, 2 out]
      }
      frame Default {
        n135 = Format Into String(initial string="Main Function ", error in=w1331, w1332) -> (resulting string=w1335:string, error out=w1330:errorcluster)  [unwired: 1 in]
        n136 = Concatenate Strings(w1335, " not defined" ("string")) -> (w1333:string)
        n137 = One Button Dialog(message=w1333) -> ()  [unwired: 1 in, 1 out]
      }
    }
    n138 = call <vilib>:"Simple Error Handler.vi"("error in (no error)"=w26) -> ("error out"=w28:errorcluster)  [unwired: 4 in, 4 out]
  }
  n139 = while {
    shift-right: [w1340] -> _
    shift-left: w8 -> [w1341]
    shift-right: [w1342] -> _
    shift-left: w7 -> [w1339]
    stop <- w1337 stop-if-true
    n140 = event shown="[46] \"MU_Calibration_getOptimizedNoniusTrackOffsetTableBaseOnly\": Value Change" {
      selector: _ -> [_ _ _ _ _ _ _ _ _ _ _ _ _ _ _ _ _ _ _ _ _ _ _ _ _ _ _ _ _ _ _ _ _ _ _ _ _ _ _ _ _ _ _ _ _ _ _ _ _ _ _ _ _ _ _ _ _ _ _ _ _ _ _ _ _ _ _ _ _ _ _ _ _ _ _ _ _ _ _ _ _ _ _ _ _ _ _ _ _ _ _ _ _ _ _ _ _ _ _ _ _ _ _ _ _ _ _ _ _ _ _ _ _ _ _ _ _ _ _ _]
      dyn-events: _ -> [_ _ _ _ _ _ _ _ _ _ _ _ _ _ _ _ _ _ _ _ _ _ _ _ _ _ _ _ _ _ _ _ _ _ _ _ _ _ _ _ _ _ _ _ _ _ _ _ _ _ _ _ _ _ _ _ _ _ _ _ _ _ _ _ _ _ _ _ _ _ _ _ _ _ _ _ _ _ _ _ _ _ _ _ _ _ _ _ _ _ _ _ _ _ _ _ _ _ _ _ _ _ _ _ _ _ _ _ _ _ _ _ _ _ _ _ _ _ _ _]
      timeout: _ -> [_ _ _ _ _ _ _ _ _ _ _ _ _ _ _ _ _ _ _ _ _ _ _ _ _ _ _ _ _ _ _ _ _ _ _ _ _ _ _ _ _ _ _ _ _ _ _ _ _ _ _ _ _ _ _ _ _ _ _ _ _ _ _ _ _ _ _ _ _ _ _ _ _ _ _ _ _ _ _ _ _ _ _ _ _ _ _ _ _ _ _ _ _ _ _ _ _ _ _ _ _ _ _ _ _ _ _ _ _ _ _ _ _ _ _ _ _ _ _ _]
      tunnel: w1339 -> [w1348 w1354 w1360 w1366 w1370 w1378 w1384 w1388 w1394 w1400 w1407 w1414 w1419 w1425 w1432 w1438 w1443 w1449 w1455 w1461 w1467 w1473 w1479 w1485 w1491 w1497 w1503 w1509 w1515 w1521 w1527 w1533 w1539 w1545 w1551 w1557 w1563 w1570 w1576 w1582 w1588 w1594 w1600 w1606 w1612 w1618 w1624 w1630 w1636 w1642 w1648 w1654 w1660 w1666 w1672 w1678 w1684 w1690 w1696 w1702 w1708 w1714 w1720 w1726 w1732 w1738 w1744 w1750 w1756 w1762 w1768 w1774 w1780 w1786 w1792 w1798 w1804 w1810 w1816 w1822 w1828 w1834 w1839 w1845 w1851 w1858 w1864 w1870 w1876 w1882 w1888 w1894 w1900 w1904 w1912 w1918 w1924 w1930 w1936 w1942 w1948 w1954 w1960 w1966 w1972 w1978 w1984 w1990 w1996 w2002 w2008 w2014 w2020 w2026 w2032 w2038 w2044 w2050 w2056 w2061]
      tunnel: [w1347 w1353 w1359 w1365 w1372 w1377 w1383 w1387 w1391 w1397 w1406 w1413 w1420 w1426 w1431 w1437 w1441 w1447 w1453 w1459 w1465 w1471 w1477 w1483 w1489 w1495 w1501 w1507 w1513 w1519 w1525 w1531 w1537 w1543 w1549 w1555 w1561 w1568 w1574 w1580 w1586 w1592 w1598 w1604 w1610 w1616 w1622 w1628 w1634 w1640 w1646 w1652 w1658 w1664 w1670 w1676 w1682 w1688 w1694 w1700 w1706 w1712 w1718 w1724 w1730 w1736 w1742 w1748 w1754 w1760 w1766 w1772 w1778 w1784 w1790 w1797 w1803 w1809 w1815 w1821 w1827 w1833 w1838 w1844 w1850 w1857 w1863 w1869 w1875 w1881 w1887 w1893 w1899 w1903 w1911 w1917 w1923 w1929 w1935 w1941 w1947 w1953 w1959 w1965 w1971 w1977 w1983 w1989 w1995 w2001 w2007 w2013 w2019 w2025 w2031 w2037 w2043 w2049 w2055 w2058] -> w1342
      tunnel: w1341 -> [w1345 w1351 w1357 w1363 w1369 w1375 w1381 w1386 w1393 w1399 w1405 w1411 w1418 w1424 w1429 w1435 w1442 w1448 w1454 w1460 w1466 w1472 w1478 w1484 w1490 w1496 w1502 w1508 w1514 w1520 w1526 w1532 w1538 w1544 w1550 w1556 w1562 w1569 w1575 w1581 w1587 w1593 w1599 w1605 w1611 w1617 w1623 w1629 w1635 w1641 w1647 w1653 w1659 w1665 w1671 w1677 w1683 w1689 w1695 w1701 w1707 w1713 w1719 w1725 w1731 w1737 w1743 w1749 w1755 w1761 w1767 w1773 w1779 w1785 w1791 w1795 w1801 w1807 w1813 w1819 w1825 w1831 w1837 w1843 w1849 w1855 w1861 w1867 w1873 w1879 w1885 w1891 w1897 w1902 w1909 w1915 w1921 w1927 w1933 w1939 w1945 w1951 w1957 w1963 w1969 w1975 w1981 w1987 w1993 w1999 w2005 w2011 w2017 w2023 w2029 w2035 w2041 w2047 w2053 w2060]
      tunnel: [w1346 w1352 w1358 w1364 w1371 w1376 w1382 w1385 w1392 w1398 w1404 w1412 w1417 w1423 w1430 w1436 w1440 w1446 w1452 w1458 w1464 w1470 w1476 w1482 w1488 w1494 w1500 w1506 w1512 w1518 w1524 w1530 w1536 w1542 w1548 w1554 w1560 w1567 w1573 w1579 w1585 w1591 w1597 w1603 w1609 w1615 w1621 w1627 w1633 w1639 w1645 w1651 w1657 w1663 w1669 w1675 w1681 w1687 w1693 w1699 w1705 w1711 w1717 w1723 w1729 w1735 w1741 w1747 w1753 w1759 w1765 w1771 w1777 w1783 w1789 w1796 w1802 w1808 w1814 w1820 w1826 w1832 w1836 w1842 w1848 w1856 w1862 w1868 w1874 w1880 w1886 w1892 w1898 w1901 w1910 w1916 w1922 w1928 w1934 w1940 w1946 w1952 w1958 w1964 w1970 w1976 w1982 w1988 w1994 w2000 w2006 w2012 w2018 w2024 w2030 w2036 w2042 w2048 w2054 w2059] -> w1340
      tunnel: FALSE -> [w1343 w1349 w1355 w1361 w1367 w1373 w1379 w1390 w1396 w1402 w1403 w1409 w1415 w1421 w1427 w1433 w1439 w1445 w1451 w1457 w1463 w1469 w1475 w1481 w1487 w1493 w1499 w1505 w1511 w1517 w1523 w1529 w1535 w1541 w1547 w1553 w1559 w1566 w1572 w1578 w1584 w1590 w1596 w1602 w1608 w1614 w1620 w1626 w1632 w1638 w1644 w1650 w1656 w1662 w1668 w1674 w1680 w1686 w1692 w1698 w1704 w1710 w1716 w1722 w1728 w1734 w1740 w1746 w1752 w1758 w1764 w1770 w1776 w1782 w1788 w1793 w1799 w1805 w1811 w1817 w1823 w1829 w1835 w1841 w1847 w1853 w1859 w1865 w1871 w1877 w1883 w1889 w1895 w1906 w1907 w1913 w1919 w1925 w1931 w1938 w1944 w1950 w1956 w1962 w1968 w1974 w1980 w1986 w1992 w1998 w2004 w2010 w2016 w2022 w2028 w2034 w2040 w2046 w2052 _]
      tunnel: [w1343 w1349 w1355 w1361 w1367 w1373 w1379 w1390 w1396 w1402 w1403 w1409 w1415 w1421 w1427 w1433 w1439 w1445 w1451 w1457 w1463 w1469 w1475 w1481 w1487 w1493 w1499 w1505 w1511 w1517 w1523 w1529 w1535 w1541 w1547 w1553 w1559 w1566 w1572 w1578 w1584 w1590 w1596 w1602 w1608 w1614 w1620 w1626 w1632 w1638 w1644 w1650 w1656 w1662 w1668 w1674 w1680 w1686 w1692 w1698 w1704 w1710 w1716 w1722 w1728 w1734 w1740 w1746 w1752 w1758 w1764 w1770 w1776 w1782 w1788 w1793 w1799 w1805 w1811 w1817 w1823 w1829 w1835 w1841 w1847 w1853 w1859 w1865 w1871 w1877 w1883 w1889 w1895 w1906 w1907 w1913 w1919 w1925 w1931 w1938 w1944 w1950 w1956 w1962 w1968 w1974 w1980 w1986 w1992 w1998 w2004 w2010 w2016 w2022 w2028 w2034 w2040 w2046 w2052 TRUE] -> w1337
      event "MU_Open": Value Change {
        n141 = event-data() -> ()  [unwired: 1 in, 1 out]
        n142 = Enqueue Element(queue=w1345, element=MU_Functions."Open" ("Events"), error in (no error)=w1348) -> (queue out=w1346:refnum<queue>, error out=w1347:errorcluster)  [unwired: 1 in, 1 out]
      }
      event "MU_Close": Value Change {
        n143 = event-data() -> ()  [unwired: 1 in, 1 out]
        n144 = Enqueue Element(queue=w1351, element=MU_Functions."Close" ("Events"), error in (no error)=w1354) -> (queue out=w1352:refnum<queue>, error out=w1353:errorcluster)  [unwired: 1 in, 1 out]
      }
      event "MU_SetInterface": Value Change {
        n145 = event-data() -> ()  [unwired: 1 in, 1 out]
        n146 = Enqueue Element(queue=w1357, element=MU_Functions."Set Interface" ("Events"), error in (no error)=w1360) -> (queue out=w1358:refnum<queue>, error out=w1359:errorcluster)  [unwired: 1 in, 1 out]
      }
      event "MU_GetInterface": Value Change {
        n147 = event-data() -> ()  [unwired: 1 in, 1 out]
        n148 = Enqueue Element(queue=w1363, element=MU_Functions."Get Interface" ("Events"), error in (no error)=w1366) -> (queue out=w1364:refnum<queue>, error out=w1365:errorcluster)  [unwired: 1 in, 1 out]
      }
      event "MU_SetConfig": Value Change {
        n149 = event-data() -> ()  [unwired: 1 in, 1 out]
        n150 = Enqueue Element(queue=w1369, element=MU_Functions."Set Config" ("Events"), error in (no error)=w1370) -> (queue out=w1371:refnum<queue>, error out=w1372:errorcluster)  [unwired: 1 in, 1 out]
      }
      event "MU_GetConfig": Value Change {
        n151 = event-data() -> ()  [unwired: 1 in, 1 out]
        n152 = Enqueue Element(queue=w1375, element=MU_Functions."Get Config" ("Events"), error in (no error)=w1378) -> (queue out=w1376:refnum<queue>, error out=w1377:errorcluster)  [unwired: 1 in, 1 out]
      }
      event "MU_SwitchToBiSS": Value Change {
        n153 = event-data() -> ()  [unwired: 1 in, 1 out]
        n154 = Enqueue Element(queue=w1381, element=MU_Functions."Switch to BiSS" ("Events"), error in (no error)=w1384) -> (queue out=w1382:refnum<queue>, error out=w1383:errorcluster)  [unwired: 1 in, 1 out]
      }
      event "MU_SwitchToBiSS_Ex": Value Change {
        n155 = event-data() -> ()  [unwired: 1 in, 1 out]
        n156 = Enqueue Element(queue=w1386, element=MU_Functions."Switch to BiSS Ex" ("Events"), error in (no error)=w1388) -> (queue out=w1385:refnum<queue>, error out=w1387:errorcluster)  [unwired: 1 in, 1 out]
      }
      event "MU_EnableGetMT": Value Change {
        n157 = event-data() -> ()  [unwired: 1 in, 1 out]
        n158 = Enqueue Element(queue=w1393, element=MU_Functions."Enable Get MT" ("Events"), error in (no error)=w1394) -> (queue out=w1392:refnum<queue>, error out=w1391:errorcluster)  [unwired: 1 in, 1 out]
      }
      event "MU_DisableGetMT": Value Change {
        n159 = event-data() -> ()  [unwired: 1 in, 1 out]
        n160 = Enqueue Element(queue=w1399, element=MU_Functions."Disable Get MT" ("Events"), error in (no error)=w1400) -> (queue out=w1398:refnum<queue>, error out=w1397:errorcluster)  [unwired: 1 in, 1 out]
      }
      event "MU_Initialize": Value Change {
        n161 = event-data() -> ()  [unwired: 1 in, 1 out]
        n162 = Enqueue Element(queue=w1405, element=MU_Functions."Initialize" ("Events"), error in (no error)=w1407) -> (queue out=w1404:refnum<queue>, error out=w1406:errorcluster)  [unwired: 1 in, 1 out]
      }
      event "MU_SetParam": Value Change {
        n163 = event-data() -> ()  [unwired: 1 in, 1 out]
        n164 = Enqueue Element(queue=w1411, element=MU_Functions."Set Param" ("Events"), error in (no error)=w1414) -> (queue out=w1412:refnum<queue>, error out=w1413:errorcluster)  [unwired: 1 in, 1 out]
      }
      event "MU_GetParam": Value Change {
        n165 = event-data() -> ()  [unwired: 1 in, 1 out]
        n166 = Enqueue Element(queue=w1418, element=MU_Functions."Get Param" ("Events"), error in (no error)=w1419) -> (queue out=w1417:refnum<queue>, error out=w1420:errorcluster)  [unwired: 1 in, 1 out]
      }
      event "MU_IsParameterAvailableInUsedRevision": Value Change {
        n167 = event-data() -> ()  [unwired: 1 in, 1 out]
        n168 = Enqueue Element(queue=w1424, element=MU_Functions."Is Parameter Available In Used Revision" ("Events"), error in (no error)=w1425) -> (queue out=w1423:refnum<queue>, error out=w1426:errorcluster)  [unwired: 1 in, 1 out]
      }
      event "MU_WriteParams": Value Change {
        n169 = event-data() -> ()  [unwired: 1 in, 1 out]
        n170 = Enqueue Element(queue=w1429, element=MU_Functions."Write Params" ("Events"), error in (no error)=w1432) -> (queue out=w1430:refnum<queue>, error out=w1431:errorcluster)  [unwired: 1 in, 1 out]
      }
      event "MU_ReadParams": Value Change {
        n171 = event-data() -> ()  [unwired: 1 in, 1 out]
        n172 = Enqueue Element(queue=w1435, element=MU_Functions."Read Params" ("Events"), error in (no error)=w1438) -> (queue out=w1436:refnum<queue>, error out=w1437:errorcluster)  [unwired: 1 in, 1 out]
      }
      event "MU_ReadStatus": Value Change {
        n173 = event-data() -> ()  [unwired: 1 in, 1 out]
        n174 = Enqueue Element(queue=w1442, element=MU_Functions."Read Status" ("Events"), error in (no error)=w1443) -> (queue out=w1440:refnum<queue>, error out=w1441:errorcluster)  [unwired: 1 in, 1 out]
      }
      event "MU_ReadGain": Value Change {
        n175 = event-data() -> ()  [unwired: 1 in, 1 out]
        n176 = Enqueue Element(queue=w1448, element=MU_Functions."Read Gain" ("Events"), error in (no error)=w1449) -> (queue out=w1446:refnum<queue>, error out=w1447:errorcluster)  [unwired: 1 in, 1 out]
      }
      event "MU_WriteEeprom": Value Change {
        n177 = event-data() -> ()  [unwired: 1 in, 1 out]
        n178 = Enqueue Element(queue=w1454, element=MU_Functions."Write Eeprom" ("Events"), error in (no error)=w1455) -> (queue out=w1452:refnum<queue>, error out=w1453:errorcluster)  [unwired: 1 in, 1 out]
      }
      event "MU_WriteCmdRegister": Value Change {
        n179 = event-data() -> ()  [unwired: 1 in, 1 out]
        n180 = Enqueue Element(queue=w1460, element=MU_Functions."Write Cmd Register" ("Events"), error in (no error)=w1461) -> (queue out=w1458:refnum<queue>, error out=w1459:errorcluster)  [unwired: 1 in, 1 out]
      }
      event "MU_WriteSwitchCommand": Value Change {
        n181 = event-data() -> ()  [unwired: 1 in, 1 out]
        n182 = Enqueue Element(queue=w1466, element=MU_Functions."Write Switch Command" ("Events"), error in (no error)=w1467) -> (queue out=w1464:refnum<queue>, error out=w1465:errorcluster)  [unwired: 1 in, 1 out]
      }
      event "MU_ReadSens": Value Change {
        n183 = event-data() -> ()  [unwired: 1 in, 1 out]
        n184 = Enqueue Element(queue=w1472, element=MU_Functions."Read Sens" ("Events"), error in (no error)=w1473) -> (queue out=w1470:refnum<queue>, error out=w1471:errorcluster)  [unwired: 1 in, 1 out]
      }
      event "MU_Get Calibration": Value Change {
        n185 = event-data() -> ()  [unwired: 1 in, 1 out]
        n186 = Enqueue Element(queue=w1478, element=MU_Functions."Get Calibration" ("Events"), error in (no error)=w1479) -> (queue out=w1476:refnum<queue>, error out=w1477:errorcluster)  [unwired: 1 in, 1 out]
      }
      event "MU_Set Calibration": Value Change {
        n187 = event-data() -> ()  [unwired: 1 in, 1 out]
        n188 = Enqueue Element(queue=w1484, element=MU_Functions."Set Calibration" ("Events"), error in (no error)=w1485) -> (queue out=w1482:refnum<queue>, error out=w1483:errorcluster)  [unwired: 1 in, 1 out]
      }
      event "MU_Calibration_setCurrentAnalogTrackAdjustments": Value Change {
        n189 = event-data() -> ()  [unwired: 1 in, 1 out]
        n190 = Enqueue Element(queue=w1490, element=MU_Functions."Calibration_setCurrentAnalogTrackAdjustments" ("Events"), error in (no error)=w1491) -> (queue out=w1488:refnum<queue>, error out=w1489:errorcluster)  [unwired: 1 in, 1 out]
      }
      event "MU_activateCalibrationConfig": Value Change {
        n191 = event-data() -> ()  [unwired: 1 in, 1 out]
        n192 = Enqueue Element(queue=w1496, element=MU_Functions."ActivateCalibrationConfig" ("Events"), error in (no error)=w1497) -> (queue out=w1494:refnum<queue>, error out=w1495:errorcluster)  [unwired: 1 in, 1 out]
      }
      event "MU_deactivateCalibrationConfig": Value Change {
        n193 = event-data() -> ()  [unwired: 1 in, 1 out]
        n194 = Enqueue Element(queue=w1502, element=MU_Functions."DeactivateCalibrationConfig" ("Events"), error in (no error)=w1503) -> (queue out=w1500:refnum<queue>, error out=w1501:errorcluster)  [unwired: 1 in, 1 out]
      }
      event "MU_Interface_nearestPossibleClockFreq": Value Change {
        n195 = event-data() -> ()  [unwired: 1 in, 6 out]
        n196 = Enqueue Element(queue=w1508, element=MU_Functions."InterfaceNearestPossibleClockFreq" ("Events"), error in (no error)=w1509) -> (queue out=w1506:refnum<queue>, error out=w1507:errorcluster)  [unwired: 1 in, 1 out]
      }
      event "MU_Interface_nearestPossibleFrameCycleTime": Value Change {
        n197 = event-data() -> ()  [unwired: 1 in, 6 out]
        n198 = Enqueue Element(queue=w1514, element=MU_Functions."InterfaceNearestPossibleFrameCycleTime" ("Events"), error in (no error)=w1515) -> (queue out=w1512:refnum<queue>, error out=w1513:errorcluster)  [unwired: 1 in, 1 out]
      }
      event "MU_Interface_nextPossibleFrameCycleTime": Value Change {
        n199 = event-data() -> ()  [unwired: 1 in, 6 out]
        n200 = Enqueue Element(queue=w1520, element=MU_Functions."InterfaceNextPossibleFrameCycleTime" ("Events"), error in (no error)=w1521) -> (queue out=w1518:refnum<queue>, error out=w1519:errorcluster)  [unwired: 1 in, 1 out]
      }
      event "MU_Interface_nextPossibleClockFreq": Value Change {
        n201 = event-data() -> ()  [unwired: 1 in, 6 out]
        n202 = Enqueue Element(queue=w1526, element=MU_Functions."InterfaceNextPossibleClockFreq" ("Events"), error in (no error)=w1527) -> (queue out=w1524:refnum<queue>, error out=w1525:errorcluster)  [unwired: 1 in, 1 out]
      }
      event "MU_generateBissIdentifier": Value Change {
        n203 = event-data() -> ()  [unwired: 1 in, 6 out]
        n204 = Enqueue Element(queue=w1532, element=MU_Functions."generateBissIdentifier" ("Events"), error in (no error)=w1533) -> (queue out=w1530:refnum<queue>, error out=w1531:errorcluster)  [unwired: 1 in, 1 out]
      }
      event "MU_generateBissProfileId": Value Change {
        n205 = event-data() -> ()  [unwired: 1 in, 6 out]
        n206 = Enqueue Element(queue=w1538, element=MU_Functions."generateBissProfileId" ("Events"), error in (no error)=w1539) -> (queue out=w1536:refnum<queue>, error out=w1537:errorcluster)  [unwired: 1 in, 1 out]
      }
      event "MU_acquireRawData": Value Change {
        n207 = event-data() -> ()  [unwired: 1 in, 6 out]
        n208 = Enqueue Element(queue=w1544, element=MU_Functions."AcquireRawData" ("Events"), error in (no error)=w1545) -> (queue out=w1542:refnum<queue>, error out=w1543:errorcluster)  [unwired: 1 in, 1 out]
      }
      event "MU_Calibration_analyzeRawData": Value Change {
        n209 = event-data() -> ()  [unwired: 1 in, 6 out]
        n210 = Enqueue Element(queue=w1550, element=MU_Functions."Calibration_AnalyzeRawData" ("Events"), error in (no error)=w1551) -> (queue out=w1548:refnum<queue>, error out=w1549:errorcluster)  [unwired: 1 in, 1 out]
      }
      event "MU_Calibration_getRelativeMasterTrackAdjustments": Value Change {
        n211 = event-data() -> ()  [unwired: 1 in, 6 out]
        n212 = Enqueue Element(queue=w1556, element=MU_Functions."Calibration_GetRelativeMasterTrackAdjustments" ("Events"), error in (no error)=w1557) -> (queue out=w1554:refnum<queue>, error out=w1555:errorcluster)  [unwired: 1 in, 1 out]
      }
      event "MU_Calibration_getRelativeNoniusTrackAdjustments": Value Change {
        n213 = event-data() -> ()  [unwired: 1 in, 6 out]
        n214 = Enqueue Element(queue=w1562, element=MU_Functions."Calibration_GetRelativeNoniusTrackAdjustment" ("Events"), error in (no error)=w1563) -> (queue out=w1560:refnum<queue>, error out=w1561:errorcluster)  [unwired: 1 in, 1 out]
      }
      event "MU_Calibration_adjustAnalogByAnalyzeResult": Value Change {
        n215 = event-data() -> ()  [unwired: 1 in, 6 out]
        n216 = Enqueue Element(queue=w1569, element=MU_Functions."Calibration_AdjustAnalogByAnalyzeResult", error in (no error)=w1570) -> (queue out=w1567:refnum<queue>, error out=w1568:errorcluster)  [unwired: 1 in, 1 out]
      }
      event "MU_CalibrationAnalyzeResult_delete": Value Change {
        n217 = event-data() -> ()  [unwired: 1 in, 6 out]
        n218 = Enqueue Element(queue=w1575, element=MU_Functions."Calibration_AnalyzeResultdelete", error in (no error)=w1576) -> (queue out=w1573:refnum<queue>, error out=w1574:errorcluster)  [unwired: 1 in, 1 out]
      }
      event "MU_Calibration_delete": Value Change {
        n219 = event-data() -> ()  [unwired: 1 in, 1 out]
        n220 = Enqueue Element(queue=w1581, element=MU_Functions."Calibration_delete", error in (no error)=w1582) -> (queue out=w1579:refnum<queue>, error out=w1580:errorcluster)  [unwired: 1 in, 1 out]
      }
      event "MU_Calibration_numberOfCalculatedMasterPeriods": Value Change {
        n221 = event-data() -> ()  [unwired: 1 in, 1 out]
        n222 = Enqueue Element(queue=w1587, element=MU_Functions."Calibration_NumberOfCalculatedMasterPeriods", error in (no error)=w1588) -> (queue out=w1585:refnum<queue>, error out=w1586:errorcluster)  [unwired: 1 in, 1 out]
      }
      event "MU_Calibration_numberOfNoniusCurveSamples": Value Change {
        n223 = event-data() -> ()  [unwired: 1 in, 1 out]
        n224 = Enqueue Element(queue=w1593, element=MU_Functions."Calibration_NumberOfNoniusCurveSamples", error in (no error)=w1594) -> (queue out=w1591:refnum<queue>, error out=w1592:errorcluster)  [unwired: 1 in, 1 out]
      }
      event "MU_Calibration_noniusPhaseError": Value Change {
        n225 = event-data() -> ()  [unwired: 1 in, 1 out]
        n226 = Enqueue Element(queue=w1599, element=MU_Functions."Calibration_NoniusPhaseError", error in (no error)=w1600) -> (queue out=w1597:refnum<queue>, error out=w1598:errorcluster)  [unwired: 1 in, 1 out]
      }
      event "MU_Calibration_noniusTrackOffsetCurve": Value Change {
        n227 = event-data() -> ()  [unwired: 1 in, 1 out]
        n228 = Enqueue Element(queue=w1605, element=MU_Functions."Calibration_NoniusTrackOffsetCurve", error in (no error)=w1606) -> (queue out=w1603:refnum<queue>, error out=w1604:errorcluster)  [unwired: 1 in, 1 out]
      }
      event "MU_Calibration_noniusPhaseMargin": Value Change {
        n229 = event-data() -> ()  [unwired: 1 in, 1 out]
        n230 = Enqueue Element(queue=w1611, element=MU_Functions."Calibration_NoniusPhaseMargin", error in (no error)=w1612) -> (queue out=w1609:refnum<queue>, error out=w1610:errorcluster)  [unwired: 1 in, 1 out]
      }
      event "MU_Calibration_getOptimizedNoniusTrackOffsetTable": Value Change {
        n231 = event-data() -> ()  [unwired: 1 in, 1 out]
        n232 = Enqueue Element(queue=w1617, element=MU_Functions."Calibration_GetOptimizedNoniusTrackOffsetTable", error in (no error)=w1618) -> (queue out=w1615:refnum<queue>, error out=w1616:errorcluster)  [unwired: 1 in, 1 out]
      }
      event "MU_Calibration_getOptimizedNoniusTrackOffsetTableBaseOnly": Value Change {
        n233 = event-data() -> ()  [unwired: 1 in, 1 out]
        n234 = Enqueue Element(queue=w1623, element=MU_Functions."Calibration_GetOptimizedNoniusTrackOffsetBaseOnly", error in (no error)=w1624) -> (queue out=w1621:refnum<queue>, error out=w1622:errorcluster)  [unwired: 1 in, 1 out]
      }
      event "MU_Calibration_setCurrentNoniusTrackOffsetTable": Value Change {
        n235 = event-data() -> ()  [unwired: 1 in, 1 out]
        n236 = Enqueue Element(queue=w1629, element=MU_Functions."Calibration_SetCurrentNoniusTrackOffsetTable", error in (no error)=w1630) -> (queue out=w1627:refnum<queue>, error out=w1628:errorcluster)  [unwired: 1 in, 1 out]
      }
      event "MU_Calibration_preconfigureNumberOfMasterPeriods": Value Change {
        n237 = event-data() -> ()  [unwired: 1 in, 1 out]
        n238 = Enqueue Element(queue=w1635, element=MU_Functions."Calibration_PreconfigureNumberOfMasterPeriods", error in (no error)=w1636) -> (queue out=w1633:refnum<queue>, error out=w1634:errorcluster)  [unwired: 1 in, 1 out]
      }
      event "MU_Calibration_noniusPhaseMarginMax": Value Change {
        n239 = event-data() -> ()  [unwired: 1 in, 1 out]
        n240 = Enqueue Element(queue=w1641, element=MU_Functions."Calibration_NoniusPhaseMarginMax", error in (no error)=w1642) -> (queue out=w1639:refnum<queue>, error out=w1640:errorcluster)  [unwired: 1 in, 1 out]
      }
      event "MU_Calibration_noniusPhaseMarginMin": Value Change {
        n241 = event-data() -> ()  [unwired: 1 in, 1 out]
        n242 = Enqueue Element(queue=w1647, element=MU_Functions."Calibration_NoniusPhaseMarginMin", error in (no error)=w1648) -> (queue out=w1645:refnum<queue>, error out=w1646:errorcluster)  [unwired: 1 in, 1 out]
      }
      event "MU_Calibration_isAnalogAnalyzeResultAdjustable": Value Change {
        n243 = event-data() -> ()  [unwired: 1 in, 1 out]
        n244 = Enqueue Element(queue=w1653, element=MU_Functions."Calibration_IsAnalogAnalyzeResultAdjustable", error in (no error)=w1654) -> (queue out=w1651:refnum<queue>, error out=w1652:errorcluster)  [unwired: 1 in, 1 out]
      }
      event "MU_Calibration_numberOfAcquiredMasterPeriods": Value Change {
        n245 = event-data() -> ()  [unwired: 1 in, 1 out]
        n246 = Enqueue Element(queue=w1659, element=MU_Functions."Calibration_NumberOfAcquiredMasterPeriods", error in (no error)=w1660) -> (queue out=w1657:refnum<queue>, error out=w1658:errorcluster)  [unwired: 1 in, 1 out]
      }
      event "MU_Calibration_numberOfAcquiredNoniusPeriods": Value Change {
        n247 = event-data() -> ()  [unwired: 1 in, 1 out]
        n248 = Enqueue Element(queue=w1665, element=MU_Functions."Calibration_NumberOfAcquiredNoniusPeriods", error in (no error)=w1666) -> (queue out=w1663:refnum<queue>, error out=w1664:errorcluster)  [unwired: 1 in, 1 out]
      }
      event "MU_activateMtSyncConfig": Value Change {
        n249 = event-data() -> ()  [unwired: 1 in, 1 out]
        n250 = Enqueue Element(queue=w1671, element=MU_Functions."ActivateMtSyncConfig", error in (no error)=w1672) -> (queue out=w1669:refnum<queue>, error out=w1670:errorcluster)  [unwired: 1 in, 1 out]
      }
      event "MU_acquireMtSyncData": Value Change {
        n251 = event-data() -> ()  [unwired: 1 in, 1 out]
        n252 = Enqueue Element(queue=w1677, element=MU_Functions."AcquireMtSyncData", error in (no error)=w1678) -> (queue out=w1675:refnum<queue>, error out=w1676:errorcluster)  [unwired: 1 in, 1 out]
      }
      event "MU_deactivateMtSyncConfig": Value Change {
        n253 = event-data() -> ()  [unwired: 1 in, 1 out]
        n254 = Enqueue Element(queue=w1683, element=MU_Functions."DeactivateMtSyncConfig", error in (no error)=w1684) -> (queue out=w1681:refnum<queue>, error out=w1682:errorcluster)  [unwired: 1 in, 1 out]
      }
      event "MU_getMtSync": Value Change {
        n255 = event-data() -> ()  [unwired: 1 in, 1 out]
        n256 = Enqueue Element(queue=w1689, element=MU_Functions."GetMtSync", error in (no error)=w1690) -> (queue out=w1687:refnum<queue>, error out=w1688:errorcluster)  [unwired: 1 in, 1 out]
      }
      event "MU_MtSync_analyzeData": Value Change {
        n257 = event-data() -> ()  [unwired: 1 in, 1 out]
        n258 = Enqueue Element(queue=w1695, element=MU_Functions."MtSync_analyzeData", error in (no error)=w1696) -> (queue out=w1693:refnum<queue>, error out=w1694:errorcluster)  [unwired: 1 in, 1 out]
      }
      event "MU_MtAnalyzeResult_optimalSpoMt": Value Change {
        n259 = event-data() -> ()  [unwired: 1 in, 1 out]
        n260 = Enqueue Element(queue=w1701, element=MU_Functions."MtAnalyzeResult_optimalSpoMt", error in (no error)=w1702) -> (queue out=w1699:refnum<queue>, error out=w1700:errorcluster)  [unwired: 1 in, 1 out]
      }
      event "MU_updateMtSync": Value Change {
        n261 = event-data() -> ()  [unwired: 1 in, 1 out]
        n262 = Enqueue Element(queue=w1707, element=MU_Functions."UpdateMtSync", error in (no error)=w1708) -> (queue out=w1705:refnum<queue>, error out=w1706:errorcluster)  [unwired: 1 in, 1 out]
      }
      event "MU_MtAnalyzeResult_delete": Value Change {
        n263 = event-data() -> ()  [unwired: 1 in, 1 out]
        n264 = Enqueue Element(queue=w1713, element=MU_Functions."MtAnalyzeResult_delete", error in (no error)=w1714) -> (queue out=w1711:refnum<queue>, error out=w1712:errorcluster)  [unwired: 1 in, 1 out]
      }
      event "MU_MtSync_delete": Value Change {
        n265 = event-data() -> ()  [unwired: 1 in, 1 out]
        n266 = Enqueue Element(queue=w1719, element=MU_Functions."MtSync_delete", error in (no error)=w1720) -> (queue out=w1717:refnum<queue>, error out=w1718:errorcluster)  [unwired: 1 in, 1 out]
      }
      event "MU_activate3TrackMtSyncConfig": Value Change {
        n267 = event-data() -> ()  [unwired: 1 in, 1 out]
        n268 = Enqueue Element(queue=w1725, element=MU_Functions."Activate3TrackMtSyncConfig", error in (no error)=w1726) -> (queue out=w1723:refnum<queue>, error out=w1724:errorcluster)  [unwired: 1 in, 1 out]
      }
      event "MU_acquire3TrackMtSyncData": Value Change {
        n269 = event-data() -> ()  [unwired: 1 in, 1 out]
        n270 = Enqueue Element(queue=w1731, element=MU_Functions."Acquire3TrackMtSyncData", error in (no error)=w1732) -> (queue out=w1729:refnum<queue>, error out=w1730:errorcluster)  [unwired: 1 in, 1 out]
      }
      event "MU_deactivate3TrackMtSyncConfig": Value Change {
        n271 = event-data() -> ()  [unwired: 1 in, 1 out]
        n272 = Enqueue Element(queue=w1737, element=MU_Functions."Deactivate3TrackMtSyncConfig", error in (no error)=w1738) -> (queue out=w1735:refnum<queue>, error out=w1736:errorcluster)  [unwired: 1 in, 1 out]
      }
      event "MU_MtAnalyzeResult_calculateOffsetError": Value Change {
        n273 = event-data() -> ()  [unwired: 1 in, 1 out]
        n274 = Enqueue Element(queue=w1743, element=MU_Functions."MtAnalyzeResult_calculateOffsetError", error in (no error)=w1744) -> (queue out=w1741:refnum<queue>, error out=w1742:errorcluster)  [unwired: 1 in, 1 out]
      }
      event "MU_Calibration_calculateNoniusPosition": Value Change {
        n275 = event-data() -> ()  [unwired: 1 in, 1 out]
        n276 = Enqueue Element(queue=w1749, element=MU_Functions."Calibration_calculateNoniusPosition", error in (no error)=w1750) -> (queue out=w1747:refnum<queue>, error out=w1748:errorcluster)  [unwired: 1 in, 1 out]
      }
      event "MU_MtSync_calculatePosition": Value Change {
        n277 = event-data() -> ()  [unwired: 1 in, 1 out]
        n278 = Enqueue Element(queue=w1755, element=MU_Functions."MtSync_calculatePosition", error in (no error)=w1756) -> (queue out=w1753:refnum<queue>, error out=w1754:errorcluster)  [unwired: 1 in, 1 out]
      }
      event "MU_MtAnalyzeResult_maxOffsetError": Value Change {
        n279 = event-data() -> ()  [unwired: 1 in, 1 out]
        n280 = Enqueue Element(queue=w1761, element=MU_Functions."MtAnalyzeResult_maxOffsetError", error in (no error)=w1762) -> (queue out=w1759:refnum<queue>, error out=w1760:errorcluster)  [unwired: 1 in, 1 out]
      }
      event "MU_MtAnalyzeResult_minOffsetError": Value Change {
        n281 = event-data() -> ()  [unwired: 1 in, 1 out]
        n282 = Enqueue Element(queue=w1767, element=MU_Functions."MtAnalyzeResult_minOffsetError", error in (no error)=w1768) -> (queue out=w1765:refnum<queue>, error out=w1766:errorcluster)  [unwired: 1 in, 1 out]
      }
      event "MU_MtAnalyzeResult_offsetErrorRangeLimit": Value Change {
        n283 = event-data() -> ()  [unwired: 1 in, 1 out]
        n284 = Enqueue Element(queue=w1773, element=MU_Functions."MtAnalyzeResult_offsetErrorRangeLimit", error in (no error)=w1774) -> (queue out=w1771:refnum<queue>, error out=w1772:errorcluster)  [unwired: 1 in, 1 out]
      }
      event "MU_MtAnalyzeResult_lowerOffsetErrorMargin": Value Change {
        n285 = event-data() -> ()  [unwired: 1 in, 1 out]
        n286 = Enqueue Element(queue=w1779, element=MU_Functions."MtAnalyzeResult_lowerOffsetErrorMargin", error in (no error)=w1780) -> (queue out=w1777:refnum<queue>, error out=w1778:errorcluster)  [unwired: 1 in, 1 out]
      }
      event "MU_MtAnalyzeResult_upperOffsetErrorMargin": Value Change {
        n287 = event-data() -> ()  [unwired: 1 in, 1 out]
        n288 = Enqueue Element(queue=w1785, element=MU_Functions."MtAnalyzeResult_upperOffsetErrorMargin", error in (no error)=w1786) -> (queue out=w1783:refnum<queue>, error out=w1784:errorcluster)  [unwired: 1 in, 1 out]
      }
      event "MU_Calibration_numberOfRevolutions": Value Change {
        n289 = event-data() -> ()  [unwired: 1 in, 1 out]
        n290 = Enqueue Element(queue=w1791, element=MU_Functions."Calibration_numberOfRevolutions", error in (no error)=w1792) -> (queue out=w1789:refnum<queue>, error out=w1790:errorcluster)  [unwired: 1 in, 1 out]
      }
      event "MU_SaveParams": Value Change {
        n291 = event-data() -> ()  [unwired: 1 in, 1 out]
        n292 = Enqueue Element(queue=w1795, element=MU_Functions."Save Params" ("Events"), error in (no error)=w1798) -> (queue out=w1796:refnum<queue>, error out=w1797:errorcluster)  [unwired: 1 in, 1 out]
      }
      event "MU_ReadChipRevisionOfParameterFile": Value Change {
        n293 = event-data() -> ()  [unwired: 1 in, 1 out]
        n294 = Enqueue Element(queue=w1801, element=MU_Functions."Read Chip Revision Of Parameter File" ("Events"), error in (no error)=w1804) -> (queue out=w1802:refnum<queue>, error out=w1803:errorcluster)  [unwired: 1 in, 1 out]
      }
      event "MU_LoadParams": Value Change {
        n295 = event-data() -> ()  [unwired: 1 in, 1 out]
        n296 = Enqueue Element(queue=w1807, element=MU_Functions."Load Params" ("Events"), error in (no error)=w1810) -> (queue out=w1808:refnum<queue>, error out=w1809:errorcluster)  [unwired: 1 in, 1 out]
      }
      event "MU_GetLastError": Value Change {
        n297 = event-data() -> ()  [unwired: 1 in, 1 out]
        n298 = Enqueue Element(queue=w1813, element=MU_Functions."Get Last Error" ("Events"), error in (no error)=w1816) -> (queue out=w1814:refnum<queue>, error out=w1815:errorcluster)  [unwired: 1 in, 1 out]
      }
      event "MU_GetDLLVersion": Value Change {
        n299 = event-data() -> ()  [unwired: 1 in, 1 out]
        n300 = Enqueue Element(queue=w1819, element=MU_Functions."Get DLL Version" ("Events"), error in (no error)=w1822) -> (queue out=w1820:refnum<queue>, error out=w1821:errorcluster)  [unwired: 1 in, 1 out]
      }
      event "MU_CalcPres_POS": Value Change {
        n301 = event-data() -> ()  [unwired: 1 in, 1 out]
        n302 = Enqueue Element(queue=w1825, element=MU_Functions."Calc PRES_POS" ("Events"), error in (no error)=w1828) -> (queue out=w1826:refnum<queue>, error out=w1827:errorcluster)  [unwired: 1 in, 1 out]
      }
      event "MU_GetPres_POS": Value Change {
        n303 = event-data() -> ()  [unwired: 1 in, 1 out]
        n304 = Enqueue Element(queue=w1831, element=MU_Functions."Get PRES_POS" ("Events"), error in (no error)=w1834) -> (queue out=w1832:refnum<queue>, error out=w1833:errorcluster)  [unwired: 1 in, 1 out]
      }
      event "MU_UseRevision": Value Change {
        n305 = event-data() -> ()  [unwired: 1 in, 1 out]
        n306 = Enqueue Element(queue=w1837, element=MU_Functions."Use Revision" ("Events"), error in (no error)=w1839) -> (queue out=w1836:refnum<queue>, error out=w1838:errorcluster)  [unwired: 1 in, 1 out]
      }
      event "MU_ValueOfUsedRevision": Value Change {
        n307 = event-data() -> ()  [unwired: 1 in, 1 out]
        n308 = Enqueue Element(queue=w1843, element=MU_Functions."Value Of Used Revision" ("Events"), error in (no error)=w1845) -> (queue out=w1842:refnum<queue>, error out=w1844:errorcluster)  [unwired: 1 in, 1 out]
      }
      event "MU_ReadChipRevision": Value Change {
        n309 = event-data() -> ()  [unwired: 1 in, 1 out]
        n310 = Enqueue Element(queue=w1849, element=MU_Functions."Read Chip Revision" ("Events"), error in (no error)=w1851) -> (queue out=w1848:refnum<queue>, error out=w1850:errorcluster)  [unwired: 1 in, 1 out]
      }
      event "MU_SetRegister": Value Change {
        n311 = event-data() -> ()  [unwired: 1 in, 1 out]
        n312 = Enqueue Element(queue=w1855, element=MU_Functions."Set Register" ("Events"), error in (no error)=w1858) -> (queue out=w1856:refnum<queue>, error out=w1857:errorcluster)  [unwired: 1 in, 1 out]
      }
      event "MU_GetRegister": Value Change {
        n313 = event-data() -> ()  [unwired: 1 in, 1 out]
        n314 = Enqueue Element(queue=w1861, element=MU_Functions."Get Register" ("Events"), error in (no error)=w1864) -> (queue out=w1862:refnum<queue>, error out=w1863:errorcluster)  [unwired: 1 in, 1 out]
      }
      event "MU_WriteRegister": Value Change {
        n315 = event-data() -> ()  [unwired: 1 in, 1 out]
        n316 = Enqueue Element(queue=w1867, element=MU_Functions."Write Register" ("Events"), error in (no error)=w1870) -> (queue out=w1868:refnum<queue>, error out=w1869:errorcluster)  [unwired: 1 in, 1 out]
      }
      event "MU_ReadRegister": Value Change {
        n317 = event-data() -> ()  [unwired: 1 in, 1 out]
        n318 = Enqueue Element(queue=w1873, element=MU_Functions."Read Register" ("Events"), error in (no error)=w1876) -> (queue out=w1874:refnum<queue>, error out=w1875:errorcluster)  [unwired: 1 in, 1 out]
      }
      event "MU_WriteRegisterSSI": Value Change {
        n319 = event-data() -> ()  [unwired: 1 in, 1 out]
        n320 = Enqueue Element(queue=w1879, element=MU_Functions."Write Register SSI" ("Events"), error in (no error)=w1882) -> (queue out=w1880:refnum<queue>, error out=w1881:errorcluster)  [unwired: 1 in, 1 out]
      }
      event "MU_SaveRegister": Value Change {
        n321 = event-data() -> ()  [unwired: 1 in, 1 out]
        n322 = Enqueue Element(queue=w1885, element=MU_Functions."Save Register" ("Events"), error in (no error)=w1888) -> (queue out=w1886:refnum<queue>, error out=w1887:errorcluster)  [unwired: 1 in, 1 out]
      }
      event "MU_LoadRegister": Value Change {
        n323 = event-data() -> ()  [unwired: 1 in, 1 out]
        n324 = Enqueue Element(queue=w1891, element=MU_Functions."Load Register" ("Events"), error in (no error)=w1894) -> (queue out=w1892:refnum<queue>, error out=w1893:errorcluster)  [unwired: 1 in, 1 out]
      }
      event "MU_SPIActivate": Value Change {
        n325 = event-data() -> ()  [unwired: 1 in, 1 out]
        n326 = Enqueue Element(queue=w1897, element=MU_Functions."Spi Activate" ("Events"), error in (no error)=w1900) -> (queue out=w1898:refnum<queue>, error out=w1899:errorcluster)  [unwired: 1 in, 1 out]
      }
      event "MU_GetInterfaceInfo": Value Change {
        n327 = event-data() -> ()  [unwired: 1 in, 1 out]
        n328 = Enqueue Element(queue=w1902, element=MU_Functions."Get Interface Info" ("Events"), error in (no error)=w1904) -> (queue out=w1901:refnum<queue>, error out=w1903:errorcluster)  [unwired: 1 in, 1 out]
      }
      event "MU_WriteRegister_I2C": Value Change {
        n329 = event-data() -> ()  [unwired: 1 in, 1 out]
        n330 = Enqueue Element(queue=w1909, element=MU_Functions."Write Register I2C" ("Events"), error in (no error)=w1912) -> (queue out=w1910:refnum<queue>, error out=w1911:errorcluster)  [unwired: 1 in, 1 out]
      }
      event "MU_WriteRegister_I2C_Ex": Value Change {
        n331 = event-data() -> ()  [unwired: 1 in, 1 out]
        n332 = Enqueue Element(queue=w1915, element=MU_Functions."Write Register I2C Ex" ("Events"), error in (no error)=w1918) -> (queue out=w1916:refnum<queue>, error out=w1917:errorcluster)  [unwired: 1 in, 1 out]
      }
      event "MU_ReadRegister_I2C": Value Change {
        n333 = event-data() -> ()  [unwired: 1 in, 1 out]
        n334 = Enqueue Element(queue=w1921, element=MU_Functions."Read Register I2C" ("Events"), error in (no error)=w1924) -> (queue out=w1922:refnum<queue>, error out=w1923:errorcluster)  [unwired: 1 in, 1 out]
      }
      event "MU_SaveRegisterEx": Value Change {
        n335 = event-data() -> ()  [unwired: 1 in, 1 out]
        n336 = Enqueue Element(queue=w1927, element=MU_Functions."Save Register Ex" ("Events"), error in (no error)=w1930) -> (queue out=w1928:refnum<queue>, error out=w1929:errorcluster)  [unwired: 1 in, 1 out]
      }
      event "MU_LoadRegisterEx": Value Change {
        n337 = event-data() -> ()  [unwired: 1 in, 1 out]
        n338 = Enqueue Element(queue=w1933, element=MU_Functions."Load Register Ex" ("Events"), error in (no error)=w1936) -> (queue out=w1934:refnum<queue>, error out=w1935:errorcluster)  [unwired: 1 in, 1 out]
      }
      event "MU_GetVersionString": Value Change {
        n339 = event-data() -> ()  [unwired: 1 in, 1 out]
        n340 = Enqueue Element(queue=w1939, element=MU_Functions."Get Version String" ("Events"), error in (no error)=w1942) -> (queue out=w1940:refnum<queue>, error out=w1941:errorcluster)  [unwired: 1 in, 1 out]
      }
      event "MU_CreateCalibration": Value Change {
        n341 = event-data() -> ()  [unwired: 1 in, 1 out]
        n342 = Enqueue Element(queue=w1945, element=MU_Functions."Calibration_createCalibration" ("Events"), error in (no error)=w1948) -> (queue out=w1946:refnum<queue>, error out=w1947:errorcluster)  [unwired: 1 in, 1 out]
      }
      event "MU_Calibration_getAnalyzeResultLog": Value Change {
        n343 = event-data() -> ()  [unwired: 1 in, 1 out]
        n344 = Enqueue Element(queue=w1951, element=MU_Functions."Calibration_getAnalyzeResultLog" ("Events"), error in (no error)=w1954) -> (queue out=w1952:refnum<queue>, error out=w1953:errorcluster)  [unwired: 1 in, 1 out]
      }
      event "MU_Calibration_minimalNumberOfSamplesPerMasterPeriod": Value Change {
        n345 = event-data() -> ()  [unwired: 1 in, 1 out]
        n346 = Enqueue Element(queue=w1957, element=MU_Functions."Calibration_minimalNumberOfSamplesPerMasterPeriod" ("Events"), error in (no error)=w1960) -> (queue out=w1958:refnum<queue>, error out=w1959:errorcluster)  [unwired: 1 in, 1 out]
      }
      event "MU_Calibration_noniusPhaseRangeLimit": Value Change {
        n347 = event-data() -> ()  [unwired: 1 in, 1 out]
        n348 = Enqueue Element(queue=w1963, element=MU_Functions."Calibration_noniusPhaseRangeLimit" ("Events"), error in (no error)=w1966) -> (queue out=w1964:refnum<queue>, error out=w1965:errorcluster)  [unwired: 1 in, 1 out]
      }
      event "MU_Calibration_noniusUpperPhaseMargin": Value Change {
        n349 = event-data() -> ()  [unwired: 1 in, 1 out]
        n350 = Enqueue Element(queue=w1969, element=MU_Functions."Calibration_noniusUpperPhaseMargin" ("Events"), error in (no error)=w1972) -> (queue out=w1970:refnum<queue>, error out=w1971:errorcluster)  [unwired: 1 in, 1 out]
      }
      event "MU_Calibration_NoniusLowerPhaseMargin": Value Change {
        n351 = event-data() -> ()  [unwired: 1 in, 1 out]
        n352 = Enqueue Element(queue=w1975, element=MU_Functions."Calibration_noniusLowerPhaseMargin" ("Events"), error in (no error)=w1978) -> (queue out=w1976:refnum<queue>, error out=w1977:errorcluster)  [unwired: 1 in, 1 out]
      }
      event "MU_Calibration_getAnalogMasterTrackAdjustments": Value Change {
        n353 = event-data() -> ()  [unwired: 1 in, 1 out]
        n354 = Enqueue Element(queue=w1981, element=MU_Functions."Calibration_getAnalogMasterTrackAdjustments" ("Events"), error in (no error)=w1984) -> (queue out=w1982:refnum<queue>, error out=w1983:errorcluster)  [unwired: 1 in, 1 out]
      }
      event "MU_Calibration_getAnalogNoniusTrackAdjustments": Value Change {
        n355 = event-data() -> ()  [unwired: 1 in, 1 out]
        n356 = Enqueue Element(queue=w1987, element=MU_Functions."Calibration_getAnalogNoniusTrackAdjustments" ("Events"), error in (no error)=w1990) -> (queue out=w1988:refnum<queue>, error out=w1989:errorcluster)  [unwired: 1 in, 1 out]
      }
      event "MU_Calibration_getNoniusTrackOffsetTable": Value Change {
        n357 = event-data() -> ()  [unwired: 1 in, 1 out]
        n358 = Enqueue Element(queue=w1993, element=MU_Functions."Calibration_getNoniusTrackOffsetTable" ("Events"), error in (no error)=w1996) -> (queue out=w1994:refnum<queue>, error out=w1995:errorcluster)  [unwired: 1 in, 1 out]
      }
      event "MU_Calibration_isAnalogAnalysesValid": Value Change {
        n359 = event-data() -> ()  [unwired: 1 in, 1 out]
        n360 = Enqueue Element(queue=w1999, element=MU_Functions."Calibration_isAnalogAnalysesValid" ("Events"), error in (no error)=w2002) -> (queue out=w2000:refnum<queue>, error out=w2001:errorcluster)  [unwired: 1 in, 1 out]
      }
      event "MU_Calibration_isNoniusAnalysesValid": Value Change {
        n361 = event-data() -> ()  [unwired: 1 in, 1 out]
        n362 = Enqueue Element(queue=w2005, element=MU_Functions."Calibration_isNoniusAnalysesValid" ("Events"), error in (no error)=w2008) -> (queue out=w2006:refnum<queue>, error out=w2007:errorcluster)  [unwired: 1 in, 1 out]
      }
      event "MU_getNoniusTrackOffsetTableParameters": Value Change {
        n363 = event-data() -> ()  [unwired: 1 in, 1 out]
        n364 = Enqueue Element(queue=w2011, element=MU_Functions."getNoniusTrackOffsetTableParameters" ("Events"), error in (no error)=w2014) -> (queue out=w2012:refnum<queue>, error out=w2013:errorcluster)  [unwired: 1 in, 1 out]
      }
      event "MU_getNoniusTrackOffsetTableByParameters": Value Change {
        n365 = event-data() -> ()  [unwired: 1 in, 1 out]
        n366 = Enqueue Element(queue=w2017, element=MU_Functions."getNoniusTrackOffsetTableByParameters" ("Events"), error in (no error)=w2020) -> (queue out=w2018:refnum<queue>, error out=w2019:errorcluster)  [unwired: 1 in, 1 out]
      }
      event "MU_GetVersionMajor": Value Change {
        n367 = event-data() -> ()  [unwired: 1 in, 1 out]
        n368 = Enqueue Element(queue=w2023, element=MU_Functions."getVersionMajor" ("Events"), error in (no error)=w2026) -> (queue out=w2024:refnum<queue>, error out=w2025:errorcluster)  [unwired: 1 in, 1 out]
      }
      event "MU_GetVersionMinor": Value Change {
        n369 = event-data() -> ()  [unwired: 1 in, 1 out]
        n370 = Enqueue Element(queue=w2029, element=MU_Functions."getVersionMinor" ("Events"), error in (no error)=w2032) -> (queue out=w2030:refnum<queue>, error out=w2031:errorcluster)  [unwired: 1 in, 1 out]
      }
      event "MU_GetVersionPatch": Value Change {
        n371 = event-data() -> ()  [unwired: 1 in, 1 out]
        n372 = Enqueue Element(queue=w2035, element=MU_Functions."getVersionPatch" ("Events"), error in (no error)=w2038) -> (queue out=w2036:refnum<queue>, error out=w2037:errorcluster)  [unwired: 1 in, 1 out]
      }
      event "MU_GetVersionBuild": Value Change {
        n373 = event-data() -> ()  [unwired: 1 in, 1 out]
        n374 = Enqueue Element(queue=w2041, element=MU_Functions."getVersionBuild" ("Events"), error in (no error)=w2044) -> (queue out=w2042:refnum<queue>, error out=w2043:errorcluster)  [unwired: 1 in, 1 out]
      }
      event "MU_GetVersionSuffixString": Value Change {
        n375 = event-data() -> ()  [unwired: 1 in, 1 out]
        n376 = Enqueue Element(queue=w2047, element=MU_Functions."getVersionSuffixString" ("Events"), error in (no error)=w2050) -> (queue out=w2048:refnum<queue>, error out=w2049:errorcluster)  [unwired: 1 in, 1 out]
      }
      event "MU_createMtSync": Value Change {
        n377 = event-data() -> ()  [unwired: 1 in, 1 out]
        n378 = Enqueue Element(queue=w2053, element=MU_Functions."createMtSync" ("Events"), error in (no error)=w2056) -> (queue out=w2054:refnum<queue>, error out=w2055:errorcluster)  [unwired: 1 in, 1 out]
      }
      event "Stop Button": Value Change {
        n379 = event-data() -> ()  [unwired: 1 in, 1 out]
        n380 = Enqueue Element At Opposite End(queue=w2060, element=MU_Functions."Stop Demo" ("Events"), error in (no error)=w2061) -> (queue out=w2059:refnum<queue>, error out=w2058:errorcluster)  [unwired: 1 in, 1 out]
      }
    }
  }
